vi "vacuum2.vi"() -> ()   [LabVIEW 2014, in "Panels.lvlib"]
uses:
  Panels.lvlib
  CSlibraries-extern/DimLVEvent/DimIndicators/DimIndicators.lvlib
  CS_Core/CSSystem/CoreLib/CoreLib.lvlib
  CSlibraries/UtilityLib/UtilityLib.valueStatus.ctl
  CSlibraries/UtilityLib/UtilityLib.lvlib
  CS_Core/CSSystem/CoreLib/CoreLib.short 2 byte array.vi
  Instance           1 15Saved   vacuum2 .vi
  Instance           2 15Saved   vacuum2 .vi
  Instance           3 15Saved   vacuum2 .vi
  Instance           4 15Saved   vacuum2 .vi
  Instance           5 15Saved   vacuum2 .vi
  CSlibraries-extern/DimLVEvent/LVDimInterface/LVDimInterface.lvlib
  CS_Core/CSSystem/CoreLib/CoreLib.string 2 byte array.vi
  CS_Core/BaseProcess/BaseProcess.descriptor string definition.ctl
  CS_Core/BaseProcess/BaseProcess.lvlib
  CS_Core/CSSystem/CoreDefs/CoreDefs.rawDataType.ctl
  CS_Core/CSSystem/CoreDefs/CoreDefs.call_type.ctl
  CSlibraries-extern/DimLVEvent/DimIndicators/DimIndicators.numericType.ctl
  CSlibraries-extern/DimLVEvent/DimIndicators/DimIndicators.numericArrayType.ctl
  CSlibraries-extern/DimLVEvent/DimIndicators/DimIndicators.anyType.ctl
panel:
  out "i ref out":refnum<vi>
  out "i ref out":refnum<vi>
  in  "BOB2TISout_MonData":T1
  in  "BOB2TISin_MonData":T1
  out "BOB2TIS":bool
  in  "FVCPIR_MonData":T1={"data"=inf, "no link"=FALSE, "quality"=1, "timeStamp"=3265900746.554}
  out "FVCPIR":dbl=inf format="%.2e"
  out "LHeLevel":dbl=inf format="%.4f"
  out "LN2Level":dbl=inf format="%.4f"
  in  "LN2Level_MonData":T1={"data"=inf, "no link"=FALSE, "quality"=1, "timeStamp"=3265900746.538}
  in  "LHeLevel_MonData":T1={"data"=inf, "no link"=FALSE, "quality"=1, "timeStamp"=3265900746.554}
  in  "call cluster in":T2={"Object"="", "Selector"="", "CallType"=enum."synchronous", "Async Object"="", "Async Selector"="", "Data Descriptor"="", "Data"=[], "Error #"=0, "Expire"=0}
  in  "ReasonForLocking_SetData":T5
  in  "call cluster in":T2={"Object"="", "Selector"="", "CallType"=enum."synchronous", "Async Object"="", "Async Selector"="", "Data Descriptor"="", "Data"=[], "Error #"=0, "Expire"=0}
  in  "Reason for locking":string
  in  "BOB6_MCP_SetData":T6={"data"=[0.0, 0.0, 0.0, 0.0], "no link"=FALSE, "quality"=1, "timeStamp"=3270208307.575}
  in  "BOB6_Pho_SetData":T6={"data"=[0.0, 0.0, 0.0, 0.0], "no link"=FALSE, "quality"=1, "timeStamp"=3270208307.575}
  in  "BOB5_MCP_SetData":T6={"data"=[0.0, 0.0, 0.0, 0.0], "no link"=FALSE, "quality"=1, "timeStamp"=3270208307.575}
  in  "BOB5_Pho_SetData":T6={"data"=[0.0, 0.0, 0.0, 0.0], "no link"=FALSE, "quality"=1, "timeStamp"=3270208307.575}
  in  "BOB3_MCP_SetData":T6={"data"=[0.0, 0.0, 0.0, 0.0], "no link"=FALSE, "quality"=1, "timeStamp"=3270208307.575}
  in  "BOB3_Pho_SetData":T6={"data"=[0.0, 0.0, 0.0, 0.0], "no link"=FALSE, "quality"=1, "timeStamp"=3270208307.591}
  in  "CB5SAFE_MonData":T1
  in  "FVAPIR_MonData":T1={"data"=inf, "no link"=FALSE, "quality"=1, "timeStamp"=3265900746.538}
  in  "FVBPIR_MonData":T1={"data"=inf, "no link"=FALSE, "quality"=1, "timeStamp"=3265900746.554}
  in  "BOB6_Pho_MonData":T1={"data"=inf, "no link"=FALSE, "quality"=1, "timeStamp"=3265900746.538}
  in  "BOB5PIR_MonData":T1={"data"=inf, "no link"=FALSE, "quality"=1, "timeStamp"=3265900746.538}
  in  "PT1PEN_MonData":T1={"data"=inf, "no link"=FALSE, "quality"=1, "timeStamp"=3265900746.538}
  in  "PT1PIR_MonData":T1={"data"=inf, "no link"=FALSE, "quality"=1, "timeStamp"=3265900746.522}
  in  "BOB6_MCP_MonData":T1={"data"=inf, "no link"=FALSE, "quality"=1, "timeStamp"=3265900746.554}
  in  "PT2PIR_MonData":T1={"data"=inf, "no link"=FALSE, "quality"=1, "timeStamp"=3265900746.569}
  in  "PT2PEN_MonData":T1={"data"=inf, "no link"=FALSE, "quality"=1, "timeStamp"=3265900746.554}
  in  "PTLN2PIR_MonData":T1={"data"=inf, "no link"=FALSE, "quality"=1, "timeStamp"=3265900746.538}
  in  "CBLN2PIR_MonData":T1={"data"=inf, "no link"=FALSE, "quality"=1, "timeStamp"=3265900746.569}
  in  "BOB2PEN_MonData":T1={"data"=inf, "no link"=FALSE, "quality"=1, "timeStamp"=3265900746.554}
  in  "BOB2PIR_MonData":T1={"data"=inf, "no link"=FALSE, "quality"=1, "timeStamp"=3265900746.538}
  in  "BOB3PEN_MonData":T1={"data"=inf, "no link"=FALSE, "quality"=1, "timeStamp"=3265900746.569}
  in  "BOB5PEN_MonData":T1={"data"=inf, "no link"=FALSE, "quality"=1, "timeStamp"=3265900746.569}
  in  "BOB5_Pho_MonData":T1={"data"=inf, "no link"=FALSE, "quality"=1, "timeStamp"=3265900746.538}
  in  "BOB5_MCP_MonData":T1={"data"=inf, "no link"=FALSE, "quality"=1, "timeStamp"=3265900746.585}
  in  "BOB4PIR_MonData":T1={"data"=inf, "no link"=FALSE, "quality"=1, "timeStamp"=3265900746.538}
  in  "BOB4PEN_MonData":T1={"data"=inf, "no link"=FALSE, "quality"=1, "timeStamp"=3265900746.554}
  in  "CB3PEN_MonData":T1={"data"=inf, "no link"=FALSE, "quality"=1, "timeStamp"=3265900746.569}
  in  "CB2PEN_MonData":T1={"data"=inf, "no link"=FALSE, "quality"=1, "timeStamp"=3265900746.522}
  in  "CB1PEN_MonData":T1={"data"=inf, "no link"=FALSE, "quality"=1, "timeStamp"=3265900746.538}
  in  "BOB3_Pho_MonData":T1={"data"=inf, "no link"=FALSE, "quality"=1, "timeStamp"=3265900746.6}
  in  "BOB3_MCP_MonData":T1={"data"=inf, "no link"=FALSE, "quality"=1, "timeStamp"=3265900746.585}
  in  "BOB3PIR_MonData":T1={"data"=inf, "no link"=FALSE, "quality"=1, "timeStamp"=3265900746.569}
  out "FVAPIR":dbl=inf format="%.2e"
  out "FVBPIR":dbl=inf format="%.2e"
  out "BOB6_Pho":dbl=inf format="%.3f"
  out "BOB6_MCP":dbl=inf format="%.3f"
  out "PT1PIR":dbl=inf format="%.2e"
  out "PT1PEN":dbl=inf format="%.2e"
  out "PT2PIR":dbl=inf format="%.2e"
  out "PT2PEN":dbl=inf format="%.2e"
  out "BOB5_Pho":dbl=inf format="%.3f"
  out "BOB5_MCP":dbl=inf format="%.3f"
  out "BOB5PIR":dbl=inf format="%.2e"
  out "BOB5PEN":dbl=inf format="%.2e"
  out "BOB4PIR":dbl=inf format="%.2e"
  out "BOB4PEN":dbl=inf format="%.2e"
  out "CB3PEN":dbl=inf format="%.2e"
  out "CB2PEN":dbl=inf format="%.2e"
  out "CB1PEN":dbl=inf format="%.2e"
  out "BOB3_Pho":dbl=inf format="%.3f"
  out "BOB3_MCP":dbl=inf format="%.3f"
  out "BOB3PIR":dbl=inf format="%.2e"
  out "BOB3PEN":dbl=inf format="%.2e"
  out "BOB2PIR":dbl=inf format="%.2e"
  out "BOB2PEN":dbl=inf format="%.2e"
  out "PTLN2PIR":dbl=inf format="%.2e"
  out "CBLN2PIR":dbl=inf format="%.2e"
  in  "LASFVAout_MonData":T1
  in  "LASFVBout_MonData":T1
  in  "LASGVSout_MonData":T1
  in  "BOB2FCout_MonData":T1
  in  "BOB2FVAout_MonData":T1
  in  "BOB2FVBout_MonData":T1
  in  "BOB2GVPout_MonData":T1
  in  "BOB2GVSout_MonData":T1
  in  "BOB2TPout_MonData":T1
  in  "TSTGVSout_MonData":T1
  in  "TSTTPout_MonData":T1
  in  "TSTFVAout_MonData":T1
  in  "TSTFVBout_MonData":T1
  in  "BOB3GVSout_MonData":T1
  in  "BOB3GVPout_MonData":T1
  in  "BOB3TPout_MonData":T1
  in  "BOB3FCout_MonData":T1
  in  "BOB3MCPout_MonData":T1
  in  "BOB3FVAout_MonData":T1
  in  "BOB3FVBout_MonData":T1
  in  "CBFVAout_MonData":T1
  in  "CBFVBout_MonData":T1
  in  "CBFVCout_MonData":T1
  in  "CB1TPout_MonData":T1
  in  "CB2TPout_MonData":T1
  in  "CB3TPout_MonData":T1
  in  "CB4TPout_MonData":T1
  in  "CB5GVSout_MonData":T1
  in  "BOB4GVSout_MonData":T1
  in  "BOB4GVPout_MonData":T1
  in  "BOB4TPout_MonData":T1
  in  "BOB4BETAout_MonData":T1
  in  "BOB4FVAout_MonData":T1
  in  "BOB4FVBout_MonData":T1
  in  "BOB5GVSout_MonData":T1
  in  "BOB5GVPout_MonData":T1
  in  "BOB5TPout_MonData":T1
  in  "BOB5FCout_MonData":T1
  in  "BOB5MCPout_MonData":T1
  in  "BOB5FVAout_MonData":T1
  in  "BOB5FVBout_MonData":T1
  in  "PT1GVPout_MonData":T1
  in  "PT1TPout_MonData":T1
  in  "PT1FVAout_MonData":T1
  in  "PT1FVBout_MonData":T1
  in  "PT2GVPout_MonData":T1
  in  "PT2TPout_MonData":T1
  in  "PT2FVAout_MonData":T1
  in  "PT2FVBout_MonData":T1
  in  "BOB2lock_SetData":T1
  in  "BOB3lock_SetData":T1
  in  "BOB4lock_SetData":T1
  in  "BOB5lock_SetData":T1
  in  "TSTlock_SetData":T1
  in  "CBlock_SetData":T1
  in  "PTlock_SetData":T1
  in  "LASlock_SetData":T1
  in  "PT2FVBin_MonData":T1
  in  "PT2FVAin_MonData":T1
  in  "PT2TPin_MonData":T1
  in  "PT2GVPin_MonData":T1
  in  "PT1FVBin_MonData":T1
  in  "PT1FVAin_MonData":T1
  in  "PT1TPin_MonData":T1
  in  "PT1GVPin_MonData":T1
  in  "BOB5FVBin_MonData":T1
  in  "BOB5FVAin_MonData":T1
  in  "BOB5MCPin_MonData":T1
  in  "BOB5FCin_MonData":T1
  in  "BOB5TPin_MonData":T1
  in  "BOB5GVPin_MonData":T1
  in  "BOB5GVSin_MonData":T1
  in  "BOB4FVBin_MonData":T1
  in  "BOB4FVAin_MonData":T1
  in  "BOB4BETAin_MonData":T1
  in  "BOB4TPin_MonData":T1
  in  "BOB4GVPin_MonData":T1
  in  "BOB4GVSin_MonData":T1
  in  "CB5GVSin_MonData":T1
  in  "CB4TPin_MonData":T1
  in  "CB3TPin_MonData":T1
  in  "CB2TPin_MonData":T1
  in  "CB1TPin_MonData":T1
  in  "CBFVCin_MonData":T1
  in  "CBFVBin_MonData":T1
  in  "CBFVAin_MonData":T1
  in  "BOB3FVBin_MonData":T1
  in  "BOB3FVAin_MonData":T1
  in  "BOB3MCPin_MonData":T1
  in  "BOB3FCin_MonData":T1
  in  "BOB3TPin_MonData":T1
  in  "BOB3GVPin_MonData":T1
  in  "BOB3GVSin_MonData":T1
  in  "TSTFVBin_MonData":T1
  in  "TSTFVAin_MonData":T1
  in  "TSTTPin_MonData":T1
  in  "TSTGVSin_MonData":T1
  in  "BOB2TPin_MonData":T1
  out "TSTlock":bool
  out "BOB3lock":bool
  out "BOB6FC":bool
  out "BOB6MCP":bool=TRUE
  out "BOB3MCP":bool
  out "BOB3FC":bool
  out "BOB2FC":bool
  out "LASlock":bool
  out "BOB2lock":bool
  out "BOB5MCP":bool
  out "BOB5FC":bool
  out "BOB4BETA":bool
  out "CBlock":bool
  out "PTlock":bool
  out "BOB5lock":bool
  out "BOB4lock":bool
  out "LASGVS":bool
  out "TSTGVS":bool
  out "BOB2GVS":bool
  out "BOB3GVS":bool
  out "BOB4GVS":bool
  out "BOB5GVS":bool
  out "BOB2GVP":bool
  out "BOB3GVP":bool
  out "CB5GVS":bool
  out "BOB4GVP":bool
  out "BOB5GVP":bool
  out "PT1GVP":bool
  out "PT2GVP":bool
  out "LASFVA":bool
  out "LASFVB":bool
  out "BOB2FVA":bool
  out "BOB2FVB":bool
  out "TSTFVA":bool
  out "TSTFVB":bool
  out "BOB3FVA":bool
  out "BOB3FVB":bool
  out "CBFVA":bool
  out "CBFVC":bool
  out "CBFVB":bool
  out "BOB4FVA":bool
  out "BOB4FVB":bool
  out "BOB5FVA":bool
  out "BOB5FVB":bool
  out "PT1FVA":bool
  out "PT1FVB":bool
  out "PT2FVA":bool
  out "PT2FVB":bool
  out "CB1TP":bool
  out "BOB3TP":bool
  out "TSTTP":bool
  out "CB2TP":bool
  out "BOB2TP":bool
  out "CB5SAFE":bool=TRUE
  out "BOB5TP":bool
  out "PT2TP":bool
  out "BOB4TP":bool
  out "PT1TP":bool
  out "CB4TP":bool
  out "CB3TP":bool
  in  "BOB2GVSin_MonData":T1
  in  "BOB2GVPin_MonData":T1
  out "i ref out":refnum<vi>
  in  "BOB2FVAin_MonData":T1
  in  "BOB2FCin_MonData":T1
  in  "LASGVSin_MonData":T1
  in  "LASFVBin_MonData":T1
  in  "LASFVAin_MonData":T1
  in  "BOB2FVBin_MonData":T1
  out "PT2FVBen":bool
  out "PT2FVAen":bool
  out "PT1FVBen":bool
  out "PT1FVAen":bool
  out "BOB5FVBen":bool
  out "BOB5FVAen":bool
  out "BOB4FVBen":bool
  out "BOB4FVAen":bool
  out "BOB3FVBen":bool
  out "BOB3FVAen":bool
  out "TSTFVBen":bool
  out "BOB2FVBen":bool
  out "TSTFVAen":bool
  out "BOB2FVAen":bool
  out "LASFVBen":bool
  out "LASFVAen":bool
  out "CBFVCen":bool
  out "CBFVBen":bool
  out "CBFVAen":bool
  out "PT2GVPen":bool
  out "PT1GVPen":bool
  out "BOB5GVPen":bool
  out "BOB4GVPen":bool
  out "BOB3GVPen":bool
  out "BOB2GVPen":bool
  out "BOB5GVSen":bool
  out "BOB4GVSen":bool
  out "BOB3GVSen":bool
  out "BOB2GVSen":bool
  out "LASGVSen":bool
  out "TSTGVSen":bool
  out "BOB2TPen":bool
  out "TSTTPen":bool
  out "BOB3TPen":bool
  out "BOB4TPen":bool
  out "BOB5TPen":bool
  out "PT1TPen":bool
  out "PT2TPen":bool
  out "CB1TPen":bool
  out "CB5GVSen":bool
  # "voltage"
  # "V"
  # "voltage"
  # "V"
  # "CB5SAFE"
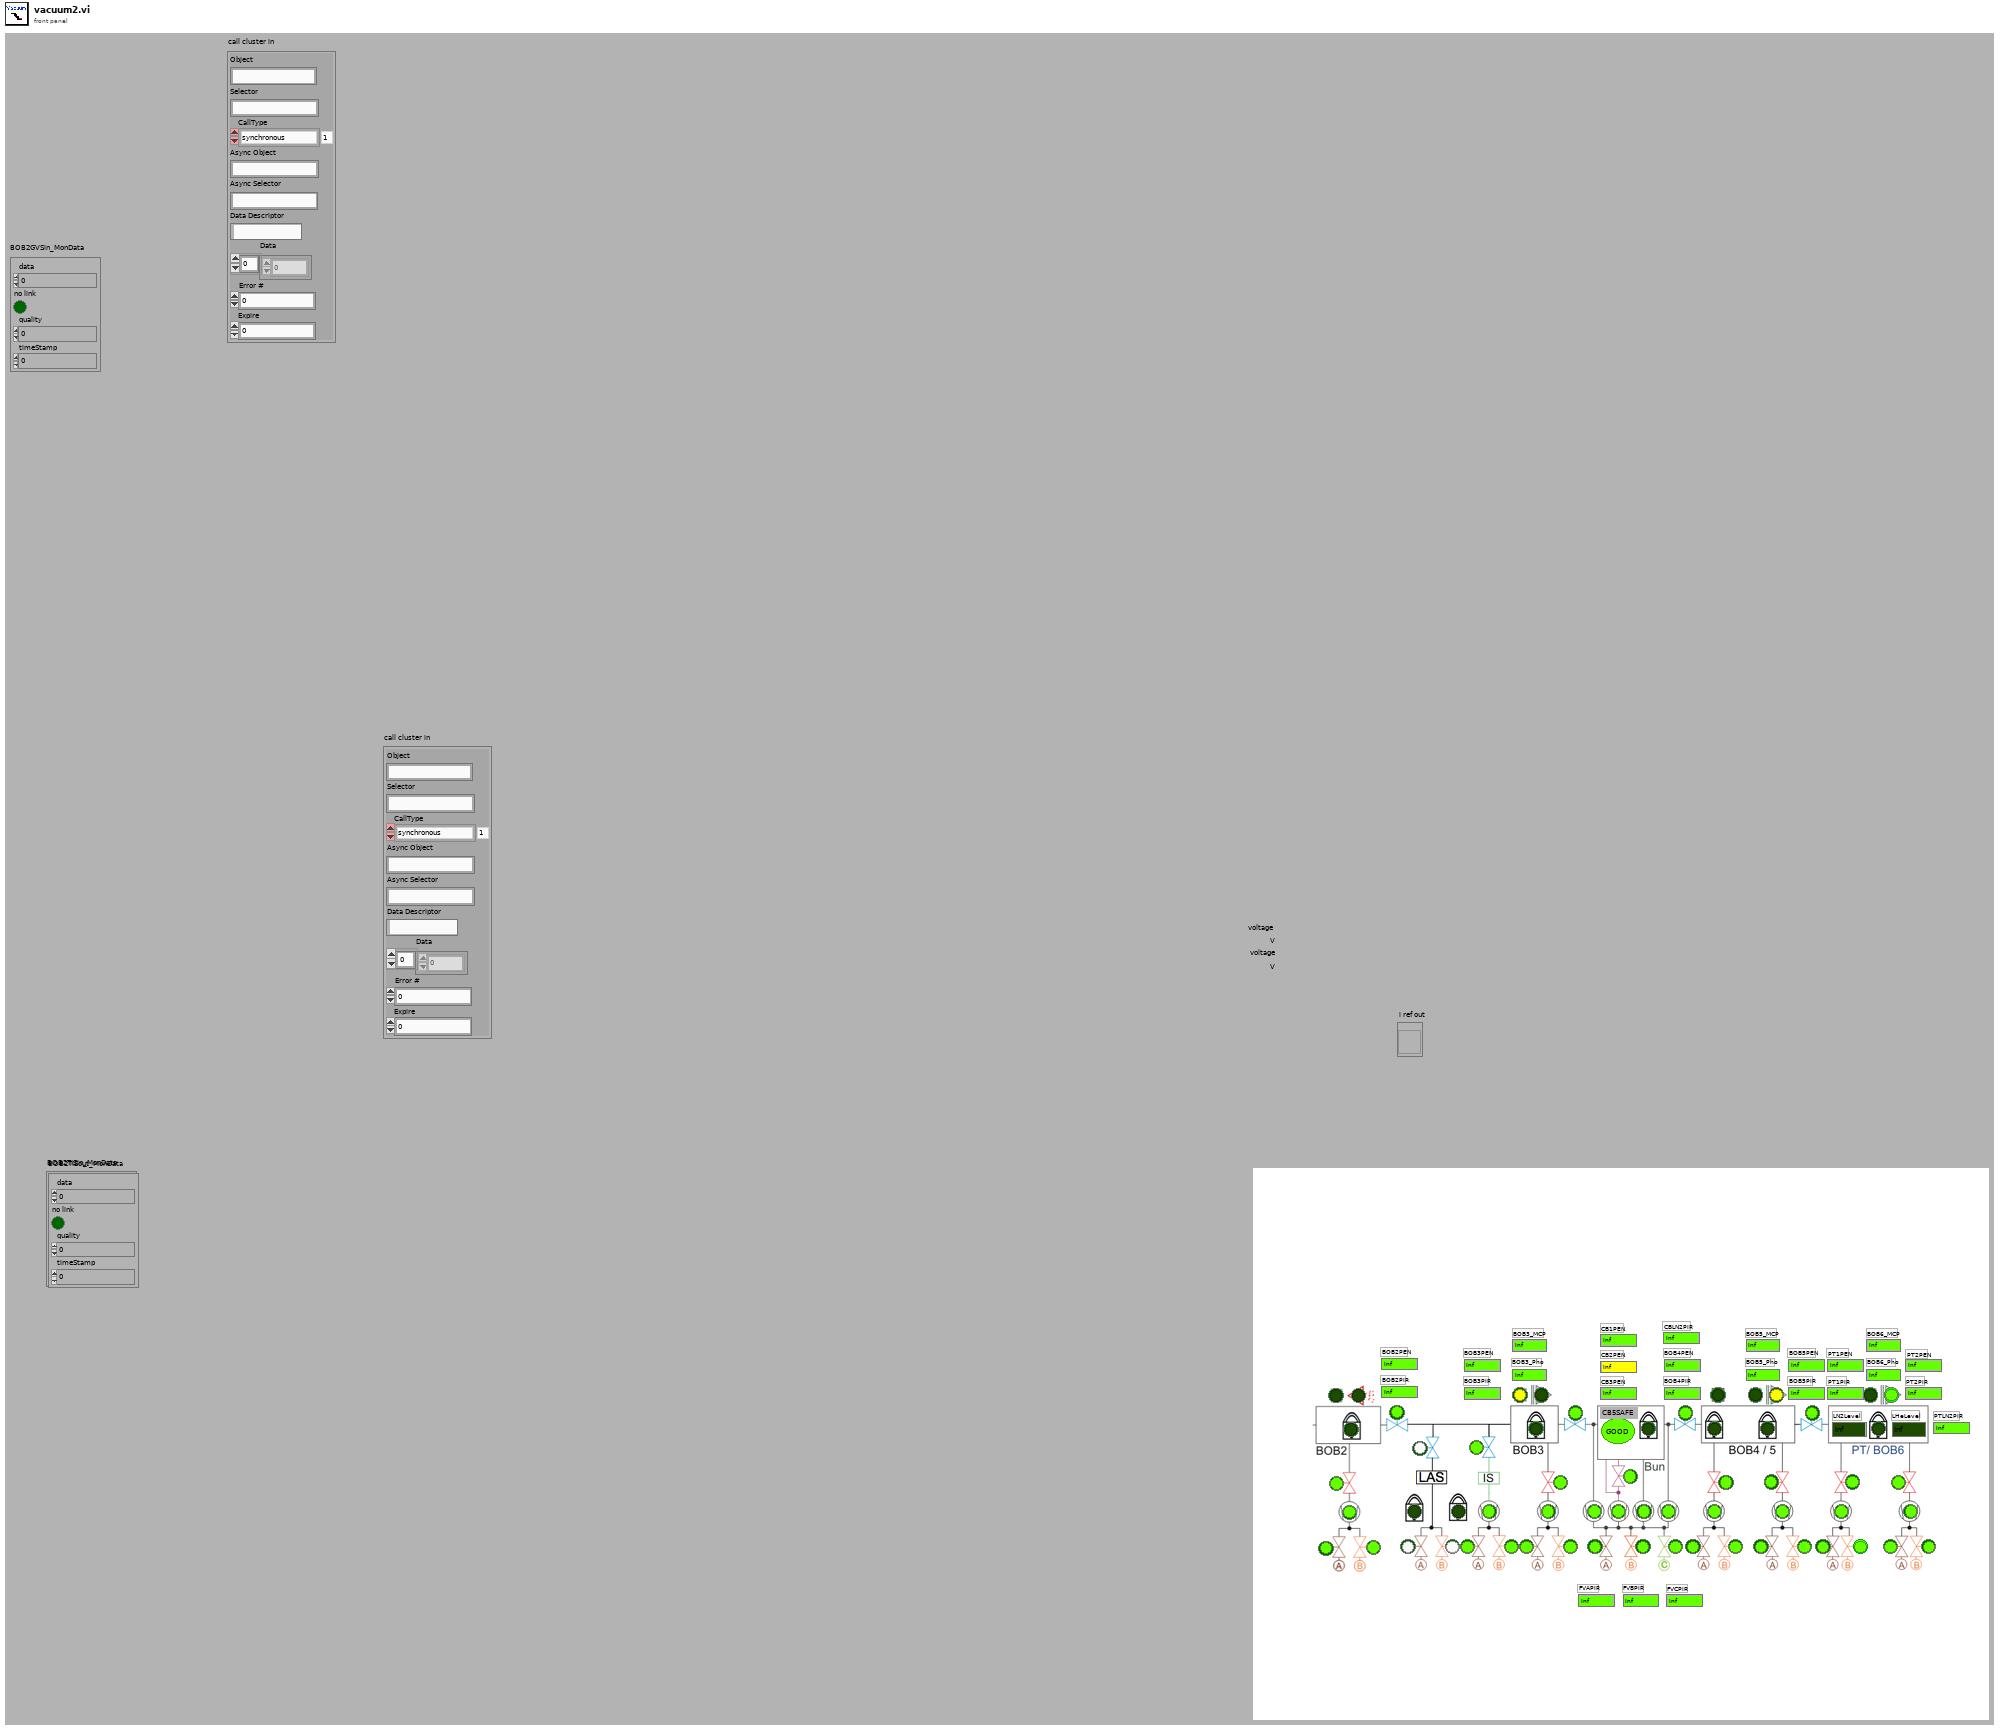
[diagram p1: front panel]
types:
  T1 = typedef "DimIndicators.lvlib/DimIndicators.numericType.ctl" = cluster{"data":dbl, "no link":bool, "quality":i32, "timeStamp":dbl}
  T2 = typedef "CoreDefs.call_type.ctl" = cluster{"Object":string, "Selector":string, "CallType":enum16{"simple", "synchronous", "asynchronous"}, "Async Object":string, "Async Selector":string, "Data Descriptor":T3, "Data":T4, "Error #":i32, "Expire":u32}
  T3 = typedef "BaseProcess.lvlib/BaseProcess.descriptor string definition.ctl" = string
  T4 = typedef "CoreDefs.rawDataType.ctl" = i8[]
  T5 = typedef "DimIndicators.lvlib/DimIndicators.anyType.ctl" = cluster{"data":string, "no link":bool, "quality":i32, "timeStamp":dbl}
  T6 = typedef "DimIndicators.lvlib/DimIndicators.numericArrayType.ctl" = cluster{"data":dbl[], "no link":bool, "quality":i32, "timeStamp":dbl}
  T7 = typedef "UtilityLib.lvlib/UtilityLib.valueStatus.ctl" = enum16{"no info available", "stand by/off", "on", "warning", "alarm/malfunction", "not implemented", "user action required", "important information", "system default", "control default", "indicator default", "button default"}
  T8 = cluster{"data":i16, "no link":bool, "quality":i32, "timeStamp":dbl}
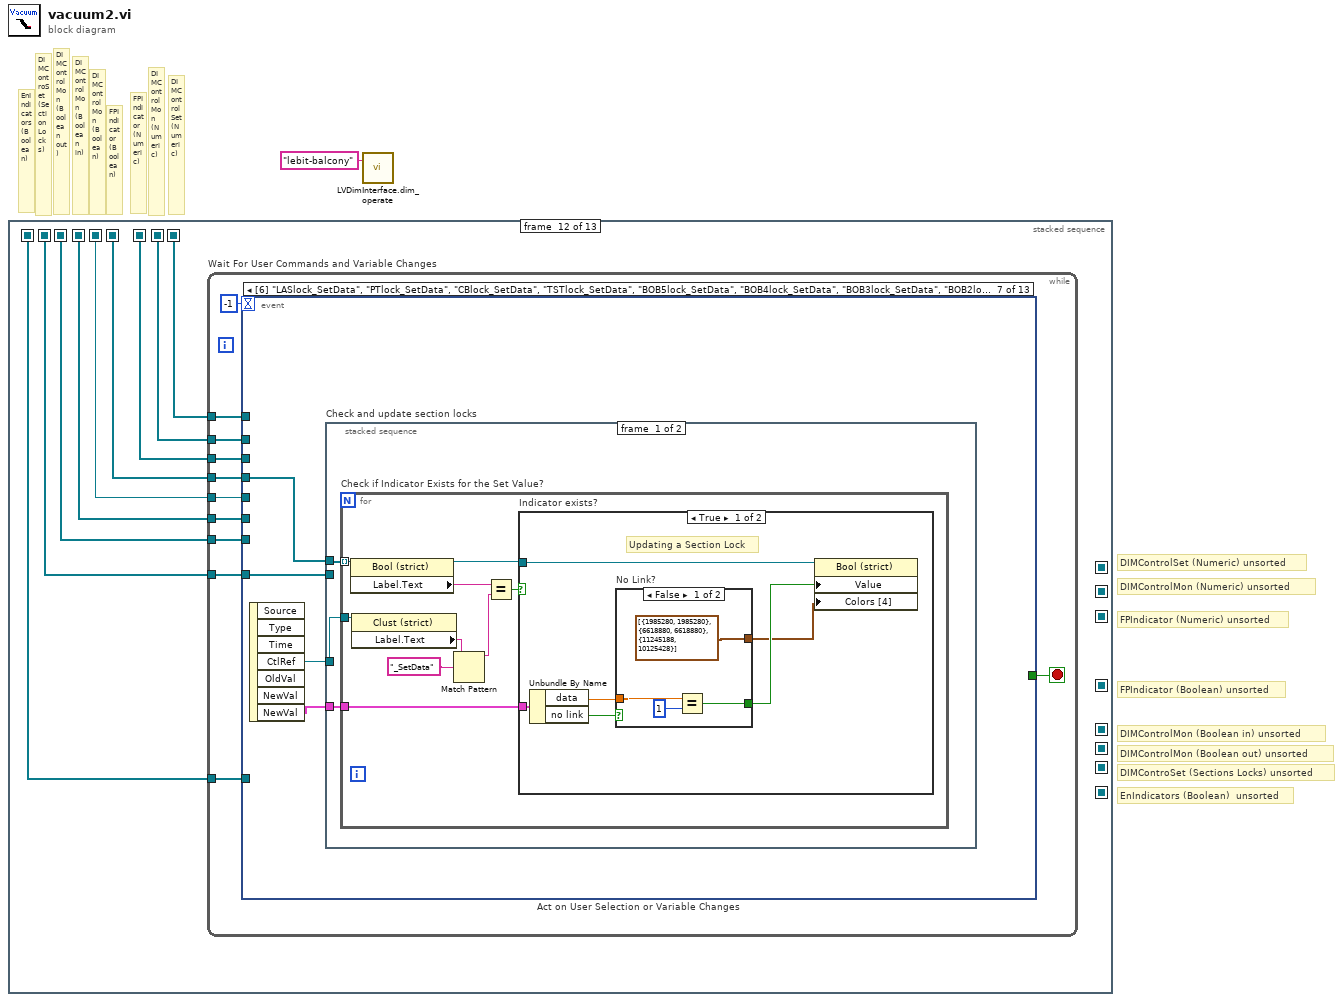
[diagram p0: block diagram]
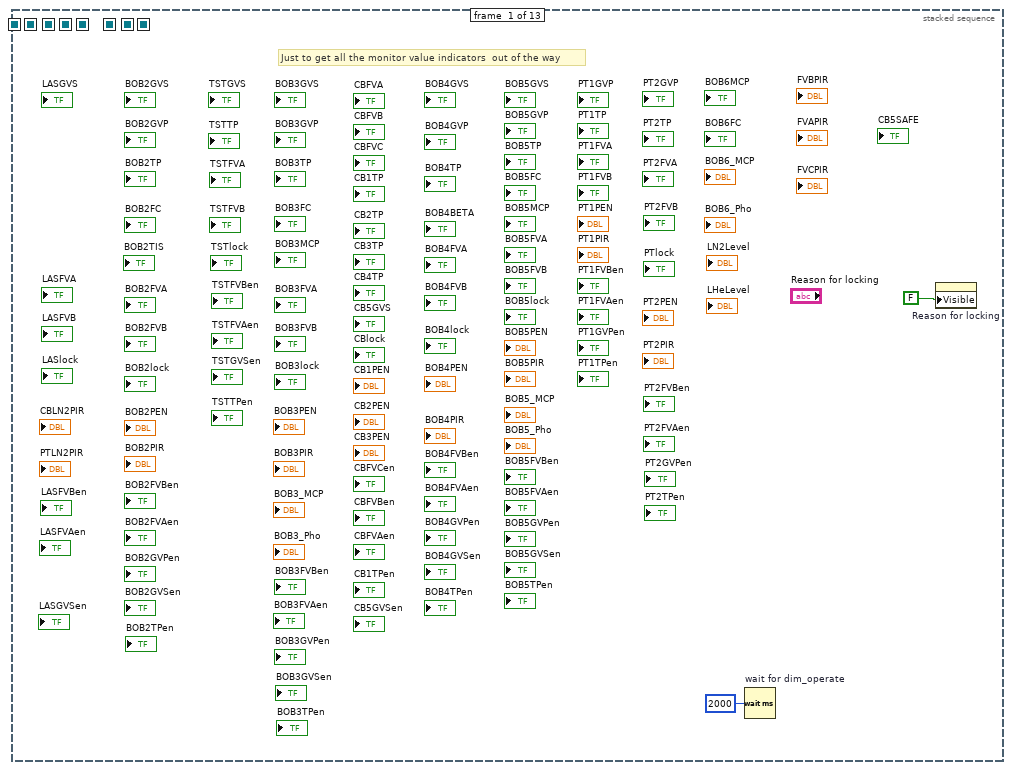
[diagram p2: hidden frame]
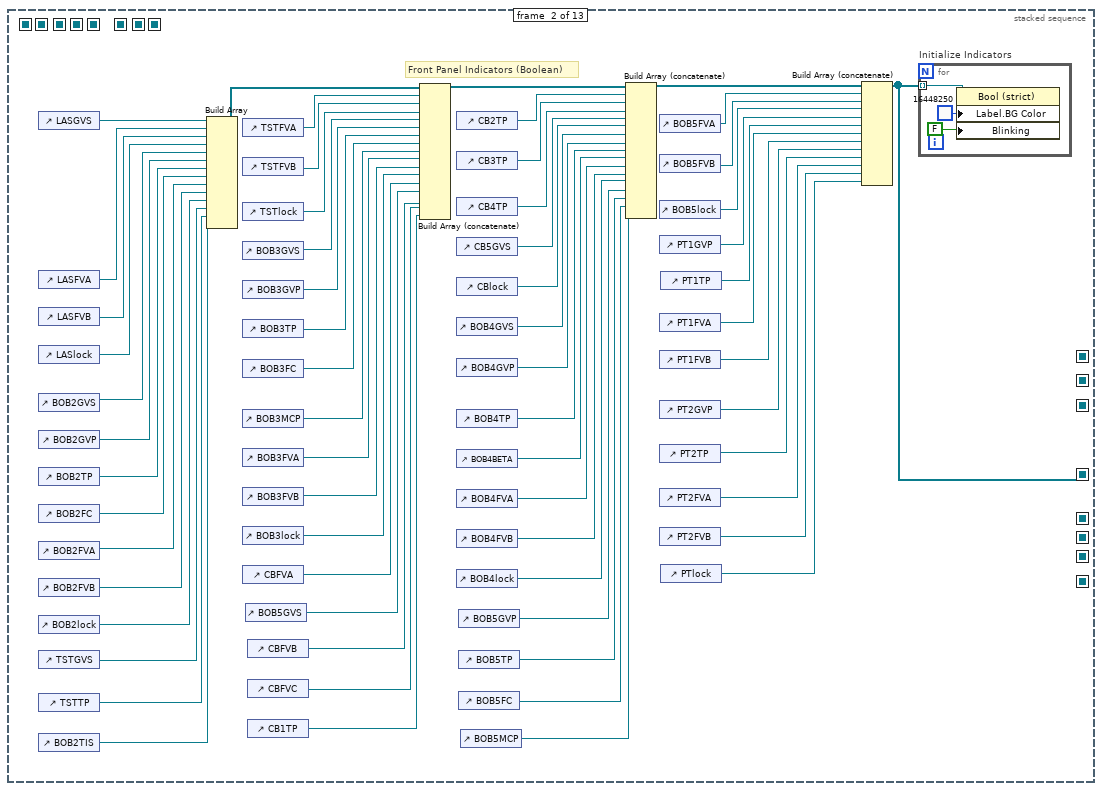
[diagram p3: hidden frame]
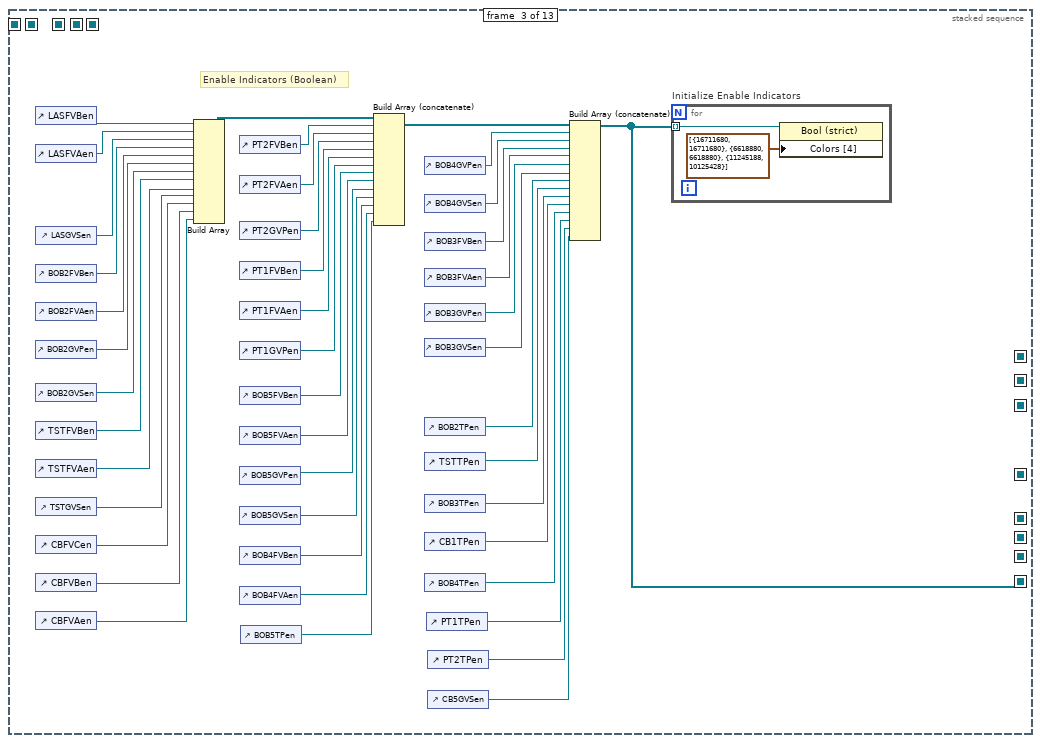
[diagram p4: hidden frame]
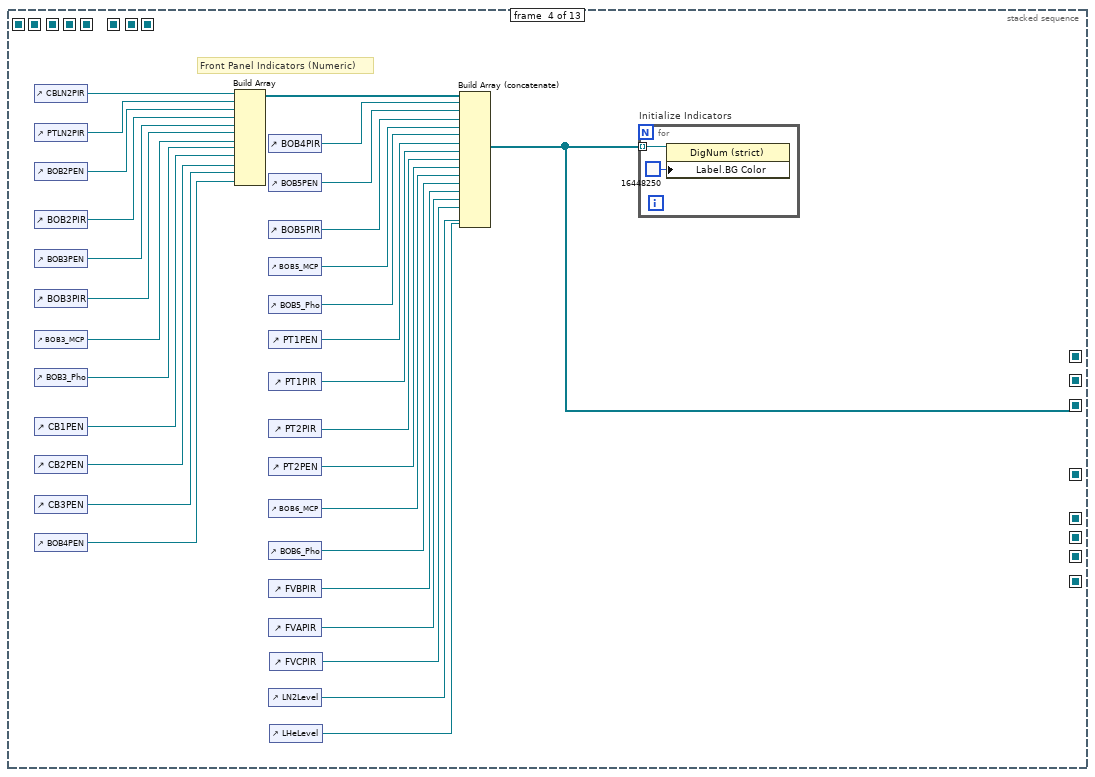
[diagram p5: hidden frame]
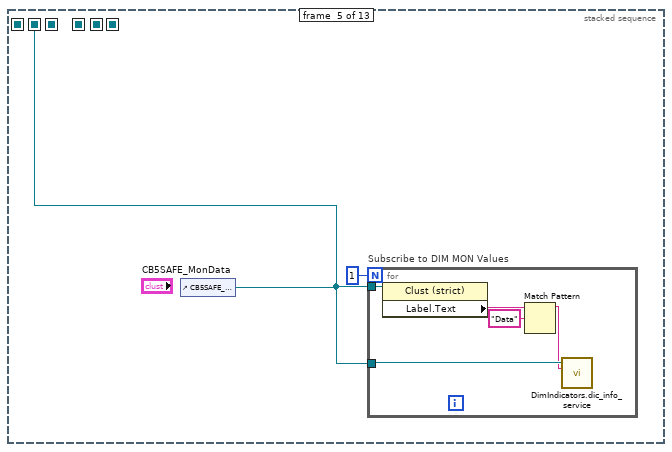
[diagram p6: hidden frame]
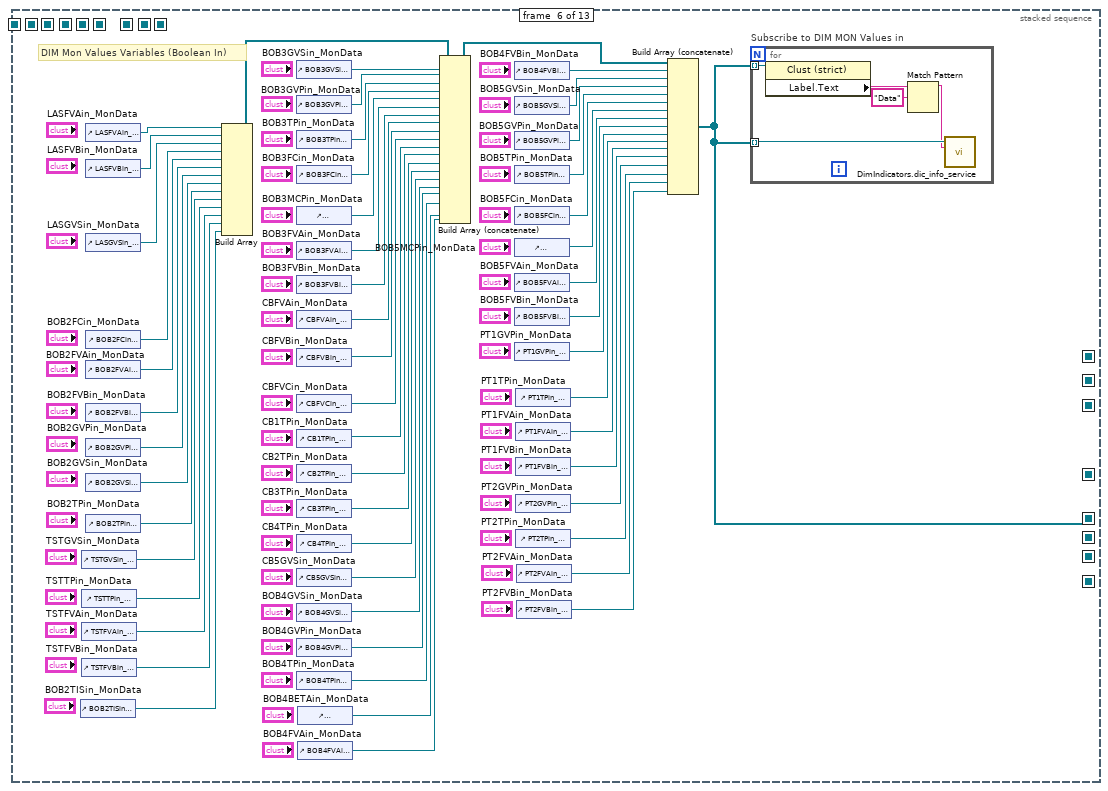
[diagram p7: hidden frame]
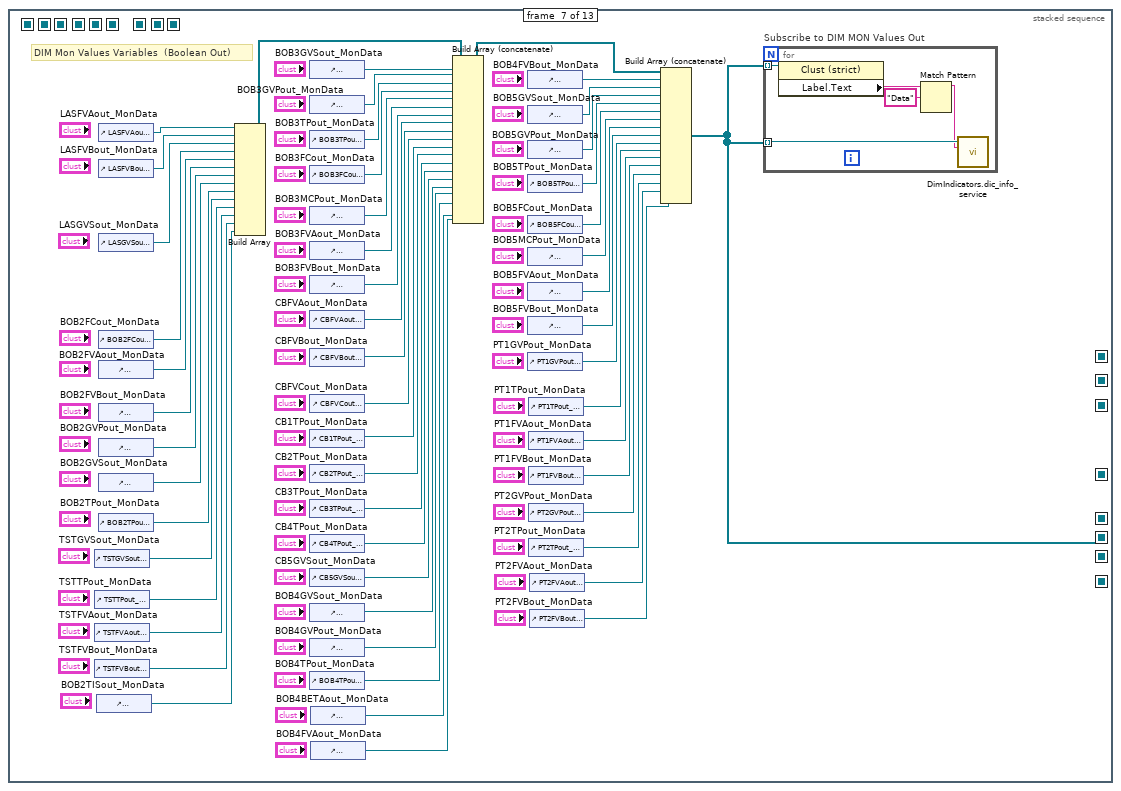
[diagram p8: hidden frame]
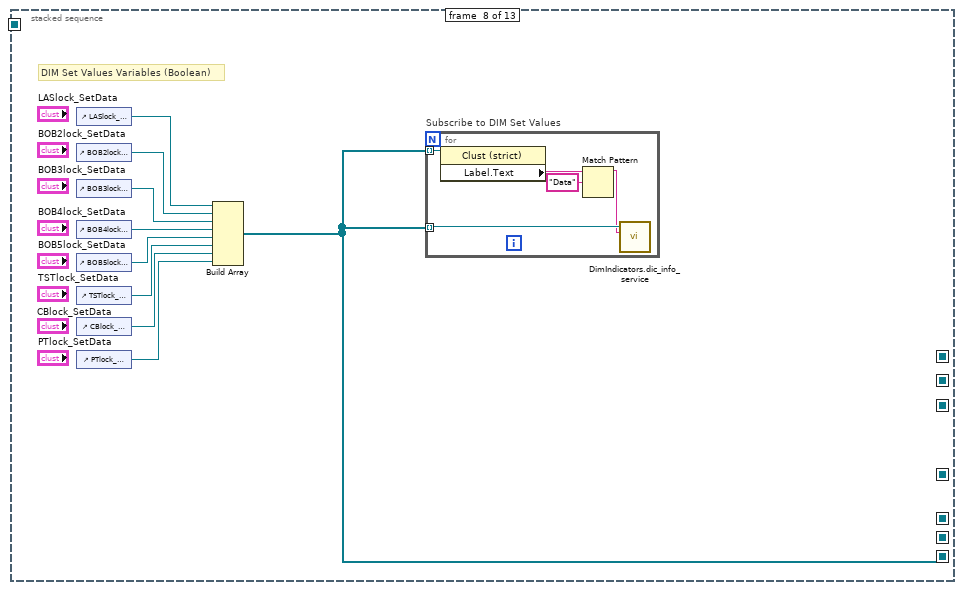
[diagram p9: hidden frame]
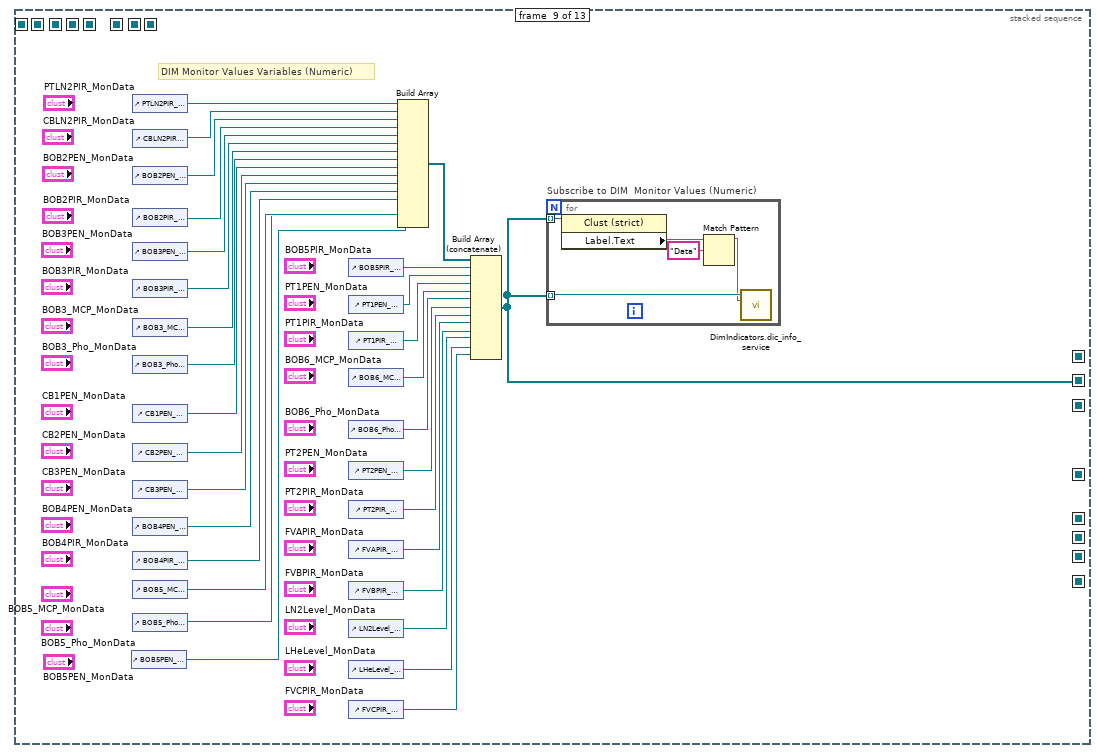
[diagram p10: hidden frame]
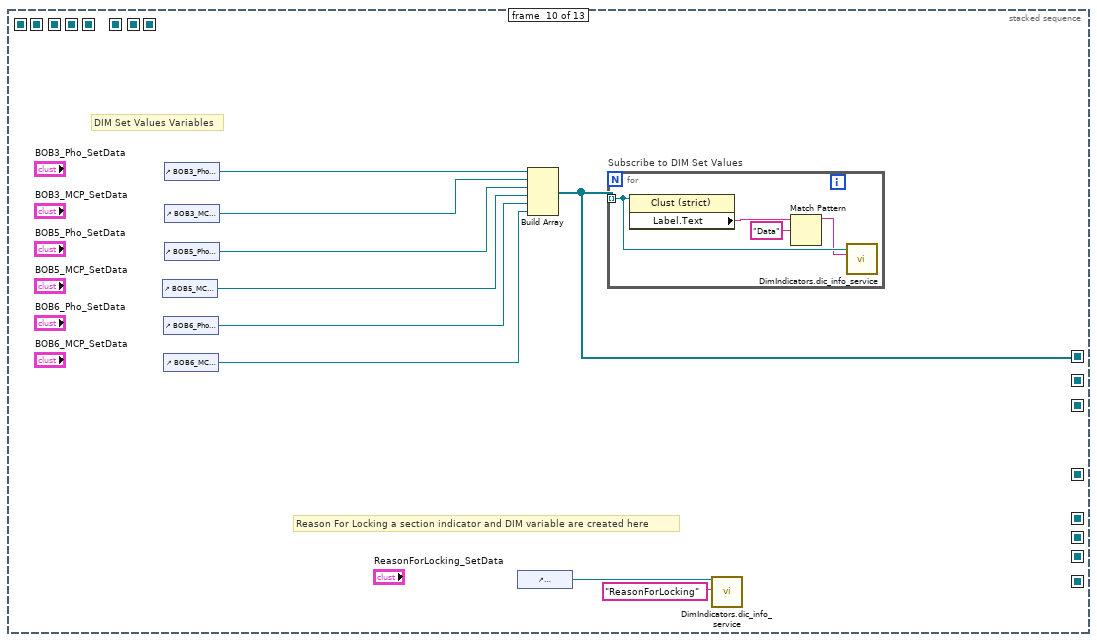
[diagram p11: hidden frame]
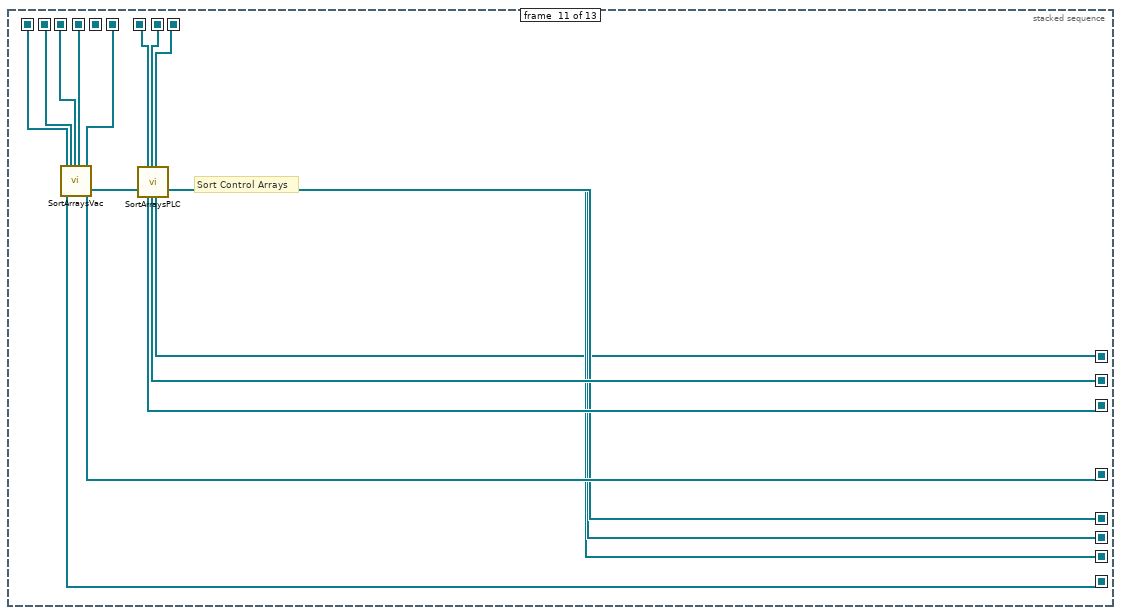
[diagram p12: hidden frame]
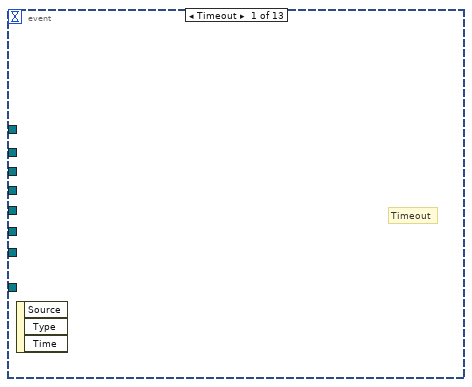
[diagram p13: hidden frame]
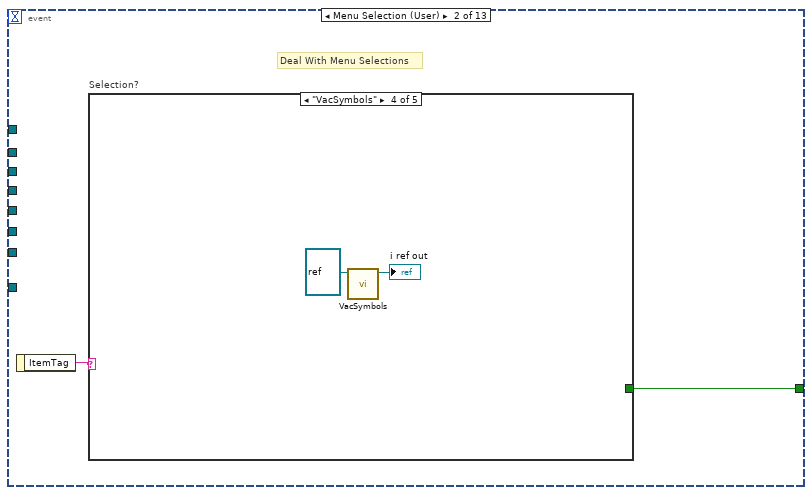
[diagram p14: hidden frame]
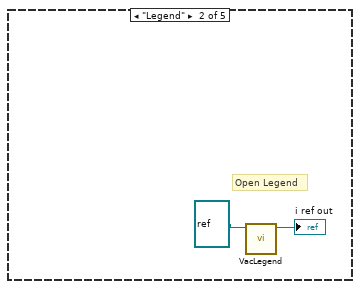
[diagram p16: hidden frame]
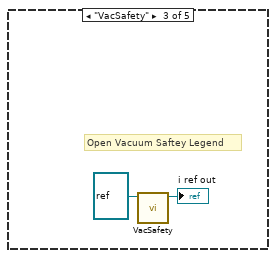
[diagram p17: hidden frame]
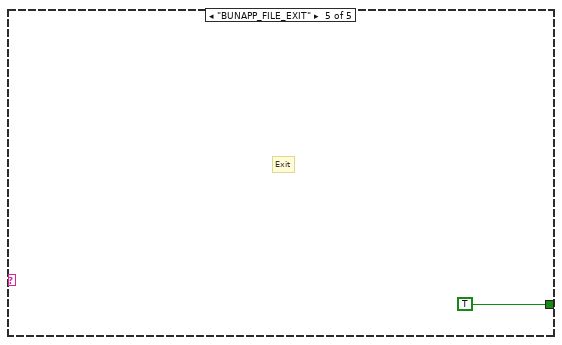
[diagram p18: hidden frame]
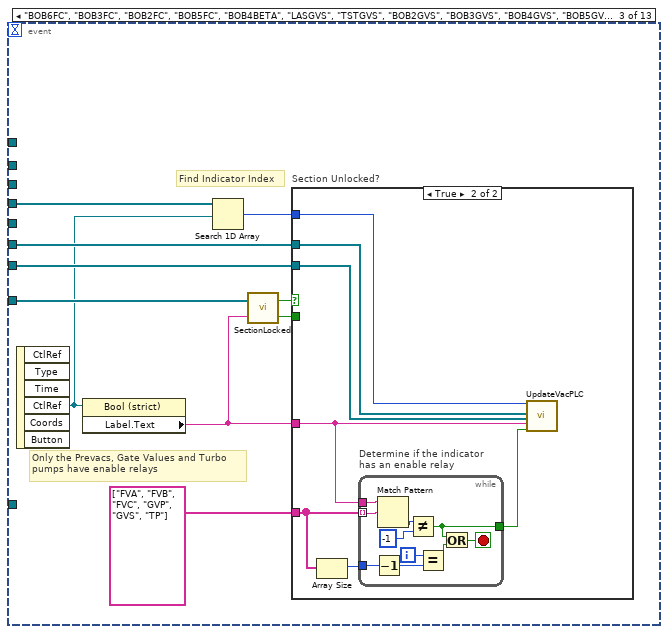
[diagram p19: hidden frame]
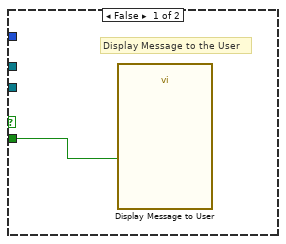
[diagram p20: hidden frame]
diagram:
  # "EnIndicators (Boolean)"
  # "EnIndicators (Boolean)  unsorted"
  # "DIMControlSet (Numeric)"
  # "DIMControlSet (Numeric) unsorted"
  # "DIMControlMon (Boolean)"
  # "DIMControlMon (Numeric) unsorted"
  # "DIMControlMon (Boolean out) unsorted"
  # "FPIndicator (Numeric) unsorted"
  # "DIMControSet (Sections Locks) unsorted"
  # "DIMControlMon (Boolean in) unsorted"
  # "FPIndicator (Boolean) unsorted"
  # "DIMControlMon (Numeric)"
  # "DIMControlMon (Boolean out)"
  # "FPIndicator (Numeric)"
  # "DIMControSet (Section Locks)"
  # "DIMControlMon (Boolean in)"
  # "FPIndicator (Boolean)"
  n1 = stacked-sequence {
    seq-local: [_ w7 _ _ _ _ _ _ _ _ _ _ _] -> [_ _ _ _ _ _ _ _ _ _ w346 _ _]
    seq-local: [_ _ _ _ _ w157 _ _ _ _ _ _ _] -> [_ _ _ _ _ _ _ _ _ _ w340 _ _]
    seq-local: [_ _ _ _ _ _ _ w269 _ _ _ _ _] -> [_ _ _ _ _ _ _ _ _ _ w338 _ _]
    seq-local: [_ _ _ w142 _ _ _ _ _ _ _ _ _] -> [_ _ _ _ _ _ _ _ _ _ w344 _ _]
    seq-local: [_ _ _ _ _ _ w215 _ _ _ _ _ _] -> [_ _ _ _ _ _ _ _ _ _ w339 _ _]
    seq-local: [_ _ _ _ _ _ _ _ w286 _ _ _ _] -> [_ _ _ _ _ _ _ _ _ _ w343 _ _]
    seq-local: [_ _ _ _ _ _ _ _ _ _ w341 _ _] -> [_ _ _ _ _ _ _ _ _ _ _ w354 w793]
    seq-local: [_ _ _ _ _ _ _ _ _ _ w337 _ _] -> [_ _ _ _ _ _ _ _ _ _ _ w351 w790]
    seq-local: [_ _ _ _ _ _ _ _ _ _ w335 _ _] -> [_ _ _ _ _ _ _ _ _ _ _ w352 w791]
    seq-local: [_ _ _ _ _ _ _ _ _ _ w336 _ _] -> [_ _ _ _ _ _ _ _ _ _ _ w353 w792]
    seq-local: [_ _ _ _ _ _ _ _ _ _ w342 _ _] -> [_ _ _ _ _ _ _ _ _ _ _ w355 _]
    seq-local: [_ _ _ _ _ _ _ _ _ _ w345 _ _] -> [_ _ _ _ _ _ _ _ _ _ _ w350 _]
    seq-local: [_ _ _ _ w147 _ _ _ _ _ _ _ _] -> [_ _ _ _ _ _ _ _ _ _ _ w349 w788]
    seq-local: [_ _ _ _ _ _ _ _ _ w320 _ _ _] -> [_ _ _ _ _ _ _ _ _ _ w334 _ _]
    seq-local: [_ _ _ _ _ _ _ _ _ _ w333 _ _] -> [_ _ _ _ _ _ _ _ _ _ _ w348 w789]
    seq-local: [_ _ w80 _ _ _ _ _ _ _ _ _ _] -> [_ _ _ _ _ _ _ _ _ _ w332 _ _]
    seq-local: [_ _ _ _ _ _ _ _ _ _ w331 _ _] -> [_ _ _ _ _ _ _ _ _ _ _ w347 _]
    frame #0 {
      # "Just to get all the monitor value indicators  out of the way"
      n2 = Wait (ms) "wait for dim_operate"(milliseconds to wait=u32 2000) -> ()  [unwired: 1 out]
      n3 = property on="Reason for locking" class="Str"("Visible"=FALSE) -> ()  [unwired: 2 in, 2 out]
    }
    frame #1 {
      # "Front Panel Indicators (Boolean)"
      # "Arrange references to all monitor-value related buttons into an array."
      n4 = control-ref of="LASGVS"() -> (w4:refnum<vi>)
      n5 = control-ref of="LASFVA"() -> (w65:refnum<vi>)
      n6 = control-ref of="LASFVB"() -> (w64:refnum<vi>)
      n7 = control-ref of="LASlock"() -> (w63:refnum<vi>)
      n8 = control-ref of="BOB2GVS"() -> (w62:refnum<vi>)
      n9 = control-ref of="BOB2GVP"() -> (w61:refnum<vi>)
      n10 = control-ref of="BOB2TP"() -> (w60:refnum<vi>)
      n11 = control-ref of="BOB2FC"() -> (w59:refnum<vi>)
      n12 = control-ref of="BOB2FVA"() -> (w58:refnum<vi>)
      n13 = control-ref of="BOB2FVB"() -> (w57:refnum<vi>)
      n14 = control-ref of="BOB2lock"() -> (w56:refnum<vi>)
      n15 = control-ref of="TSTGVS"() -> (w55:refnum<vi>)
      n16 = control-ref of="TSTTP"() -> (w54:refnum<vi>)
      n17 = control-ref of="BOB2TIS"() -> (w5:refnum<vi>)
      n18 = Build Array(w4, w65, w64, w63, w62, w61, w60, w59, w58, w57, w56, w55, w54, w5) -> (w53:refnum<vi>[])
      n19 = control-ref of="TSTFVA"() -> (w52:refnum<vi>)
      n20 = control-ref of="TSTFVB"() -> (w51:refnum<vi>)
      n21 = control-ref of="TSTlock"() -> (w50:refnum<vi>)
      n22 = control-ref of="BOB3GVS"() -> (w49:refnum<vi>)
      n23 = control-ref of="BOB3GVP"() -> (w48:refnum<vi>)
      n24 = control-ref of="BOB3TP"() -> (w47:refnum<vi>)
      n25 = control-ref of="BOB3FC"() -> (w46:refnum<vi>)
      n26 = control-ref of="BOB3MCP"() -> (w45:refnum<vi>)
      n27 = control-ref of="BOB3FVA"() -> (w44:refnum<vi>)
      n28 = control-ref of="BOB3FVB"() -> (w43:refnum<vi>)
      n29 = control-ref of="BOB3lock"() -> (w42:refnum<vi>)
      n30 = control-ref of="CBFVA"() -> (w41:refnum<vi>)
      n31 = control-ref of="BOB5GVS"() -> (w40:refnum<vi>)
      n32 = control-ref of="CBFVB"() -> (w39:refnum<vi>)
      n33 = control-ref of="CBFVC"() -> (w38:refnum<vi>)
      n34 = control-ref of="CB1TP"() -> (w37:refnum<vi>)
      n35 = Build Array (concatenate)(w53, w52, w51, w50, w49, w48, w47, w46, w45, w44, w43, w42, w41, w40, w39, w38, w37) -> (w36:refnum<vi>[])
      n36 = control-ref of="CB2TP"() -> (w35:refnum<vi>)
      n37 = control-ref of="CB3TP"() -> (w34:refnum<vi>)
      n38 = control-ref of="CB4TP"() -> (w33:refnum<vi>)
      n39 = control-ref of="CB5GVS"() -> (w32:refnum<vi>)
      n40 = control-ref of="CBlock"() -> (w31:refnum<vi>)
      n41 = control-ref of="BOB4GVS"() -> (w30:refnum<vi>)
      n42 = control-ref of="BOB4GVP"() -> (w29:refnum<vi>)
      n43 = control-ref of="BOB4TP"() -> (w28:refnum<vi>)
      n44 = control-ref of="BOB4BETA"() -> (w27:refnum<vi>)
      n45 = control-ref of="BOB4FVA"() -> (w26:refnum<vi>)
      n46 = control-ref of="BOB4FVB"() -> (w25:refnum<vi>)
      n47 = control-ref of="BOB4lock"() -> (w24:refnum<vi>)
      n48 = control-ref of="BOB5GVP"() -> (w23:refnum<vi>)
      n49 = control-ref of="BOB5TP"() -> (w22:refnum<vi>)
      n50 = control-ref of="BOB5FC"() -> (w21:refnum<vi>)
      n51 = control-ref of="BOB5MCP"() -> (w20:refnum<vi>)
      n52 = Build Array (concatenate)(w36, w35, w34, w33, w32, w31, w30, w29, w28, w27, w26, w25, w24, w23, w22, w21, w20) -> (w19:refnum<vi>[])
      n53 = control-ref of="BOB5FVA"() -> (w18:refnum<vi>)
      n54 = control-ref of="BOB5FVB"() -> (w17:refnum<vi>)
      n55 = control-ref of="BOB5lock"() -> (w16:refnum<vi>)
      n56 = control-ref of="PT1GVP"() -> (w15:refnum<vi>)
      n57 = control-ref of="PT1FVA"() -> (w14:refnum<vi>)
      n58 = control-ref of="PT1FVB"() -> (w13:refnum<vi>)
      n59 = control-ref of="PT2GVP"() -> (w12:refnum<vi>)
      n60 = control-ref of="PT2TP"() -> (w11:refnum<vi>)
      n61 = control-ref of="PT2FVA"() -> (w10:refnum<vi>)
      n62 = control-ref of="PT2FVB"() -> (w9:refnum<vi>)
      n63 = control-ref of="PT1TP"() -> (w6:refnum<vi>)
      n64 = control-ref of="PTlock"() -> (w8:refnum<vi>)
      n65 = Build Array (concatenate)(w19, w18, w17, w16, w15, w6, w14, w13, w12, w11, w10, w9, w8) -> (w7:refnum<vi>[])
      n66 = for "Initialize Indicators" {
        tunnel: w7 -> [w68] mode=indexing
        n67 = property class="Bool (strict)"(reference=w68, "Label.BG Color"=u32 16448250 ("Color Box"), "Blinking"=FALSE) -> ()  [unwired: 1 in, 2 out]
      }
    }
    frame #2 {
      # "Enable Indicators (Boolean)"
      n68 = control-ref of="LASFVBen"() -> (w69:refnum<vi>)
      n69 = control-ref of="LASFVAen"() -> (w70:refnum<vi>)
      n70 = control-ref of="LASGVSen"() -> (w111:refnum<vi>)
      n71 = control-ref of="BOB2FVBen"() -> (w110:refnum<vi>)
      n72 = control-ref of="BOB2FVAen"() -> (w109:refnum<vi>)
      n73 = control-ref of="BOB2GVPen"() -> (w108:refnum<vi>)
      n74 = control-ref of="BOB2GVSen"() -> (w107:refnum<vi>)
      n75 = control-ref of="TSTFVBen"() -> (w106:refnum<vi>)
      n76 = control-ref of="TSTFVAen"() -> (w105:refnum<vi>)
      n77 = control-ref of="TSTGVSen"() -> (w104:refnum<vi>)
      n78 = control-ref of="CBFVCen"() -> (w103:refnum<vi>)
      n79 = control-ref of="CBFVBen"() -> (w102:refnum<vi>)
      n80 = control-ref of="CBFVAen"() -> (w101:refnum<vi>)
      n81 = Build Array(w69, w70, w111, w110, w109, w108, w107, w106, w105, w104, w103, w102, w101) -> (w100:refnum<vi>[])
      n82 = control-ref of="PT2FVBen"() -> (w99:refnum<vi>)
      n83 = control-ref of="PT2FVAen"() -> (w98:refnum<vi>)
      n84 = control-ref of="PT2GVPen"() -> (w97:refnum<vi>)
      n85 = control-ref of="PT1FVBen"() -> (w96:refnum<vi>)
      n86 = control-ref of="PT1FVAen"() -> (w95:refnum<vi>)
      n87 = control-ref of="PT1GVPen"() -> (w94:refnum<vi>)
      n88 = control-ref of="BOB5FVBen"() -> (w93:refnum<vi>)
      n89 = control-ref of="BOB5FVAen"() -> (w92:refnum<vi>)
      n90 = control-ref of="BOB5GVPen"() -> (w91:refnum<vi>)
      n91 = control-ref of="BOB5GVSen"() -> (w90:refnum<vi>)
      n92 = control-ref of="BOB4FVBen"() -> (w89:refnum<vi>)
      n93 = control-ref of="BOB4FVAen"() -> (w88:refnum<vi>)
      n94 = control-ref of="BOB5TPen"() -> (w79:refnum<vi>)
      n95 = Build Array (concatenate)(w100, w99, w98, w97, w96, w95, w94, w93, w92, w91, w90, w89, w88, w79) -> (w87:refnum<vi>[])
      n96 = control-ref of="BOB4GVPen"() -> (w86:refnum<vi>)
      n97 = control-ref of="BOB4GVSen"() -> (w85:refnum<vi>)
      n98 = control-ref of="BOB3FVBen"() -> (w84:refnum<vi>)
      n99 = control-ref of="BOB3FVAen"() -> (w83:refnum<vi>)
      n100 = control-ref of="BOB3GVPen"() -> (w82:refnum<vi>)
      n101 = control-ref of="BOB3GVSen"() -> (w81:refnum<vi>)
      n102 = control-ref of="BOB2TPen"() -> (w78:refnum<vi>)
      n103 = control-ref of="TSTTPen"() -> (w77:refnum<vi>)
      n104 = control-ref of="BOB3TPen"() -> (w76:refnum<vi>)
      n105 = control-ref of="CB1TPen"() -> (w75:refnum<vi>)
      n106 = control-ref of="BOB4TPen"() -> (w74:refnum<vi>)
      n107 = control-ref of="PT1TPen"() -> (w73:refnum<vi>)
      n108 = control-ref of="PT2TPen"() -> (w72:refnum<vi>)
      n109 = control-ref of="CB5GVSen"() -> (w71:refnum<vi>)
      n110 = Build Array (concatenate)(w87, w86, w85, w84, w83, w82, w81, w78, w77, w76, w75, w74, w73, w72, w71) -> (w80:refnum<vi>[])
      n111 = for "Initialize Enable Indicators" {
        tunnel: w80 -> [w113] mode=indexing
        n112 = property class="Bool (strict)"(reference=w113, "Colors [4]"=cluster{u32, u32}[] [{16711680, 16711680}, {6618880, 6618880}, {11245188, 10125428}]) -> ()  [unwired: 1 in, 2 out]
      }
    }
    frame #3 {
      # "Front Panel Indicators (Numeric)"
      n113 = control-ref of="CBLN2PIR"() -> (w141:refnum<vi>)
      n114 = control-ref of="PTLN2PIR"() -> (w140:refnum<vi>)
      n115 = control-ref of="BOB2PEN"() -> (w139:refnum<vi>)
      n116 = control-ref of="BOB2PIR"() -> (w138:refnum<vi>)
      n117 = control-ref of="BOB3PEN"() -> (w137:refnum<vi>)
      n118 = control-ref of="BOB3PIR"() -> (w136:refnum<vi>)
      n119 = control-ref of="BOB3_MCP"() -> (w135:refnum<vi>)
      n120 = control-ref of="BOB3_Pho"() -> (w134:refnum<vi>)
      n121 = control-ref of="CB1PEN"() -> (w133:refnum<vi>)
      n122 = control-ref of="CB2PEN"() -> (w132:refnum<vi>)
      n123 = control-ref of="CB3PEN"() -> (w131:refnum<vi>)
      n124 = control-ref of="BOB4PEN"() -> (w130:refnum<vi>)
      n125 = Build Array(w141, w140, w139, w138, w137, w136, w135, w134, w133, w132, w131, w130) -> (w143:refnum<vi>[])
      n126 = control-ref of="BOB4PIR"() -> (w129:refnum<vi>)
      n127 = control-ref of="BOB5PEN"() -> (w128:refnum<vi>)
      n128 = control-ref of="BOB5PIR"() -> (w127:refnum<vi>)
      n129 = control-ref of="BOB5_MCP"() -> (w126:refnum<vi>)
      n130 = control-ref of="BOB5_Pho"() -> (w125:refnum<vi>)
      n131 = control-ref of="PT1PEN"() -> (w124:refnum<vi>)
      n132 = control-ref of="PT1PIR"() -> (w123:refnum<vi>)
      n133 = control-ref of="PT2PIR"() -> (w122:refnum<vi>)
      n134 = control-ref of="PT2PEN"() -> (w117:refnum<vi>)
      n135 = control-ref of="BOB6_MCP"() -> (w118:refnum<vi>)
      n136 = control-ref of="BOB6_Pho"() -> (w119:refnum<vi>)
      n137 = control-ref of="FVBPIR"() -> (w120:refnum<vi>)
      n138 = control-ref of="FVAPIR"() -> (w121:refnum<vi>)
      n139 = control-ref of="LN2Level"() -> (w115:refnum<vi>)
      n140 = control-ref of="FVCPIR"() -> (w116:refnum<vi>)
      n141 = control-ref of="LHeLevel"() -> (w114:refnum<vi>)
      n142 = Build Array (concatenate)(w143, w129, w128, w127, w126, w125, w124, w123, w122, w117, w118, w119, w120, w121, w116, w115, w114) -> (w142:refnum<vi>[])
      n143 = for "Initialize Indicators" {
        tunnel: w142 -> [w145] mode=indexing
        n144 = property class="DigNum (strict)"(reference=w145, "Label.BG Color"=u32 16448250 ("Color Box")) -> ()  [unwired: 1 in, 2 out]
      }
    }
    frame #4 {
      n145 = control-ref of="CB5SAFE_MonData"() -> (w147:refnum<vi>)
      n146 = for "Subscribe to DIM MON Values" {
        N: 1 -> [_]
        tunnel: w147 -> [w148]
        tunnel: w147 -> [w152]
        n147 = property class="Clust (strict)"(reference=w148) -> ("Label.Text"=w151:string)  [unwired: 1 in, 2 out]
        n148 = Match Pattern(string=w151, regular expression="Data") -> (before substring=w149:string)  [unwired: 1 in, 3 out]
        n149 = call "DimIndicators.dic_info_service.vi"("controlRef"=w152, "serviceName"=w149) -> ()  [unwired: 16 in, 2 out]
      }
    }
    frame #5 {
      # "DIM Mon Values Variables (Boolean In)"
      n150 = control-ref of="BOB2TISin_MonData"() -> (w156:refnum<vi>)
      n151 = control-ref of="TSTGVSin_MonData"() -> (w199:refnum<vi>)
      n152 = control-ref of="TSTTPin_MonData"() -> (w198:refnum<vi>)
      n153 = control-ref of="TSTFVAin_MonData"() -> (w197:refnum<vi>)
      n154 = control-ref of="TSTFVBin_MonData"() -> (w196:refnum<vi>)
      n155 = control-ref of="LASFVAin_MonData"() -> (w153:refnum<vi>)
      n156 = control-ref of="LASFVBin_MonData"() -> (w154:refnum<vi>)
      n157 = control-ref of="LASGVSin_MonData"() -> (w155:refnum<vi>)
      n158 = control-ref of="BOB2FCin_MonData"() -> (w205:refnum<vi>)
      n159 = control-ref of="BOB2FVAin_MonData"() -> (w204:refnum<vi>)
      n160 = control-ref of="BOB2FVBin_MonData"() -> (w203:refnum<vi>)
      n161 = control-ref of="BOB2GVPin_MonData"() -> (w202:refnum<vi>)
      n162 = control-ref of="BOB2GVSin_MonData"() -> (w201:refnum<vi>)
      n163 = control-ref of="BOB2TPin_MonData"() -> (w200:refnum<vi>)
      n164 = Build Array(w153, w154, w155, w205, w204, w203, w202, w201, w200, w199, w198, w197, w196, w156) -> (w194:refnum<vi>[])
      n165 = control-ref of="BOB3GVSin_MonData"() -> (w195:refnum<vi>)
      n166 = control-ref of="BOB3GVPin_MonData"() -> (w193:refnum<vi>)
      n167 = control-ref of="BOB3TPin_MonData"() -> (w192:refnum<vi>)
      n168 = control-ref of="BOB3FCin_MonData"() -> (w191:refnum<vi>)
      n169 = control-ref of="BOB3MCPin_MonData"() -> (w190:refnum<vi>)
      n170 = control-ref of="BOB3FVAin_MonData"() -> (w189:refnum<vi>)
      n171 = control-ref of="BOB3FVBin_MonData"() -> (w188:refnum<vi>)
      n172 = control-ref of="CBFVAin_MonData"() -> (w187:refnum<vi>)
      n173 = control-ref of="CBFVBin_MonData"() -> (w186:refnum<vi>)
      n174 = control-ref of="CBFVCin_MonData"() -> (w185:refnum<vi>)
      n175 = control-ref of="CB1TPin_MonData"() -> (w184:refnum<vi>)
      n176 = control-ref of="CB2TPin_MonData"() -> (w183:refnum<vi>)
      n177 = control-ref of="CB3TPin_MonData"() -> (w182:refnum<vi>)
      n178 = control-ref of="CB4TPin_MonData"() -> (w181:refnum<vi>)
      n179 = control-ref of="CB5GVSin_MonData"() -> (w180:refnum<vi>)
      n180 = control-ref of="BOB4GVSin_MonData"() -> (w179:refnum<vi>)
      n181 = control-ref of="BOB4GVPin_MonData"() -> (w178:refnum<vi>)
      n182 = control-ref of="BOB4TPin_MonData"() -> (w177:refnum<vi>)
      n183 = control-ref of="BOB4BETAin_MonData"() -> (w176:refnum<vi>)
      n184 = control-ref of="BOB4FVAin_MonData"() -> (w175:refnum<vi>)
      n185 = Build Array (concatenate)(w194, w195, w193, w192, w191, w190, w189, w188, w187, w186, w185, w184, w183, w182, w181, w180, w179, w178, w177, w176, w175) -> (w174:refnum<vi>[])
      n186 = control-ref of="BOB4FVBin_MonData"() -> (w173:refnum<vi>)
      n187 = control-ref of="BOB5GVSin_MonData"() -> (w172:refnum<vi>)
      n188 = control-ref of="BOB5GVPin_MonData"() -> (w171:refnum<vi>)
      n189 = control-ref of="BOB5TPin_MonData"() -> (w170:refnum<vi>)
      n190 = control-ref of="BOB5FCin_MonData"() -> (w169:refnum<vi>)
      n191 = control-ref of="BOB5MCPin_MonData"() -> (w168:refnum<vi>)
      n192 = control-ref of="BOB5FVAin_MonData"() -> (w167:refnum<vi>)
      n193 = control-ref of="BOB5FVBin_MonData"() -> (w166:refnum<vi>)
      n194 = control-ref of="PT1GVPin_MonData"() -> (w165:refnum<vi>)
      n195 = control-ref of="PT1TPin_MonData"() -> (w164:refnum<vi>)
      n196 = control-ref of="PT1FVAin_MonData"() -> (w163:refnum<vi>)
      n197 = control-ref of="PT1FVBin_MonData"() -> (w162:refnum<vi>)
      n198 = control-ref of="PT2GVPin_MonData"() -> (w161:refnum<vi>)
      n199 = control-ref of="PT2TPin_MonData"() -> (w160:refnum<vi>)
      n200 = control-ref of="PT2FVAin_MonData"() -> (w159:refnum<vi>)
      n201 = control-ref of="PT2FVBin_MonData"() -> (w158:refnum<vi>)
      n202 = Build Array (concatenate)(w174, w173, w172, w171, w170, w169, w168, w167, w166, w165, w164, w163, w162, w161, w160, w159, w158) -> (w157:refnum<vi>[])
      n203 = for "Subscribe to DIM MON Values in" {
        tunnel: w157 -> [w206] mode=indexing
        tunnel: w157 -> [w210] mode=indexing
        n204 = property class="Clust (strict)"(reference=w206) -> ("Label.Text"=w209:string)  [unwired: 1 in, 2 out]
        n205 = Match Pattern(string=w209, regular expression="Data") -> (before substring=w207:string)  [unwired: 1 in, 3 out]
        n206 = call "DimIndicators.dic_info_service.vi"("controlRef"=w210, "serviceName"=w207) -> ()  [unwired: 16 in, 2 out]
      }
    }
    frame #6 {
      # "DIM Mon Values Variables  (Boolean Out)"
      n207 = control-ref of="TSTGVSout_MonData"() -> (w257:refnum<vi>)
      n208 = control-ref of="TSTTPout_MonData"() -> (w256:refnum<vi>)
      n209 = control-ref of="TSTFVAout_MonData"() -> (w255:refnum<vi>)
      n210 = control-ref of="TSTFVBout_MonData"() -> (w254:refnum<vi>)
      n211 = control-ref of="BOB2TISout_MonData"() -> (w214:refnum<vi>)
      n212 = control-ref of="LASFVAout_MonData"() -> (w211:refnum<vi>)
      n213 = control-ref of="LASFVBout_MonData"() -> (w212:refnum<vi>)
      n214 = control-ref of="LASGVSout_MonData"() -> (w213:refnum<vi>)
      n215 = control-ref of="BOB2FCout_MonData"() -> (w263:refnum<vi>)
      n216 = control-ref of="BOB2FVAout_MonData"() -> (w262:refnum<vi>)
      n217 = control-ref of="BOB2FVBout_MonData"() -> (w261:refnum<vi>)
      n218 = control-ref of="BOB2GVPout_MonData"() -> (w260:refnum<vi>)
      n219 = control-ref of="BOB2GVSout_MonData"() -> (w259:refnum<vi>)
      n220 = control-ref of="BOB2TPout_MonData"() -> (w258:refnum<vi>)
      n221 = Build Array(w211, w212, w213, w263, w262, w261, w260, w259, w258, w257, w256, w255, w254, w214) -> (w252:refnum<vi>[])
      n222 = control-ref of="BOB3GVSout_MonData"() -> (w253:refnum<vi>)
      n223 = control-ref of="BOB3GVPout_MonData"() -> (w251:refnum<vi>)
      n224 = control-ref of="BOB3TPout_MonData"() -> (w250:refnum<vi>)
      n225 = control-ref of="BOB3FCout_MonData"() -> (w249:refnum<vi>)
      n226 = control-ref of="BOB3MCPout_MonData"() -> (w248:refnum<vi>)
      n227 = control-ref of="BOB3FVAout_MonData"() -> (w247:refnum<vi>)
      n228 = control-ref of="BOB3FVBout_MonData"() -> (w246:refnum<vi>)
      n229 = control-ref of="CBFVAout_MonData"() -> (w245:refnum<vi>)
      n230 = control-ref of="CBFVBout_MonData"() -> (w244:refnum<vi>)
      n231 = control-ref of="CBFVCout_MonData"() -> (w243:refnum<vi>)
      n232 = control-ref of="CB1TPout_MonData"() -> (w242:refnum<vi>)
      n233 = control-ref of="CB2TPout_MonData"() -> (w241:refnum<vi>)
      n234 = control-ref of="CB3TPout_MonData"() -> (w240:refnum<vi>)
      n235 = control-ref of="CB4TPout_MonData"() -> (w239:refnum<vi>)
      n236 = control-ref of="CB5GVSout_MonData"() -> (w238:refnum<vi>)
      n237 = control-ref of="BOB4GVSout_MonData"() -> (w237:refnum<vi>)
      n238 = control-ref of="BOB4GVPout_MonData"() -> (w236:refnum<vi>)
      n239 = control-ref of="BOB4TPout_MonData"() -> (w235:refnum<vi>)
      n240 = control-ref of="BOB4BETAout_MonData"() -> (w234:refnum<vi>)
      n241 = control-ref of="BOB4FVAout_MonData"() -> (w233:refnum<vi>)
      n242 = Build Array (concatenate)(w252, w253, w251, w250, w249, w248, w247, w246, w245, w244, w243, w242, w241, w240, w239, w238, w237, w236, w235, w234, w233) -> (w232:refnum<vi>[])
      n243 = control-ref of="BOB4FVBout_MonData"() -> (w231:refnum<vi>)
      n244 = control-ref of="BOB5GVSout_MonData"() -> (w230:refnum<vi>)
      n245 = control-ref of="BOB5GVPout_MonData"() -> (w229:refnum<vi>)
      n246 = control-ref of="BOB5TPout_MonData"() -> (w228:refnum<vi>)
      n247 = control-ref of="BOB5FCout_MonData"() -> (w227:refnum<vi>)
      n248 = control-ref of="BOB5MCPout_MonData"() -> (w226:refnum<vi>)
      n249 = control-ref of="BOB5FVAout_MonData"() -> (w225:refnum<vi>)
      n250 = control-ref of="BOB5FVBout_MonData"() -> (w224:refnum<vi>)
      n251 = control-ref of="PT1GVPout_MonData"() -> (w223:refnum<vi>)
      n252 = control-ref of="PT1TPout_MonData"() -> (w222:refnum<vi>)
      n253 = control-ref of="PT1FVAout_MonData"() -> (w221:refnum<vi>)
      n254 = control-ref of="PT1FVBout_MonData"() -> (w220:refnum<vi>)
      n255 = control-ref of="PT2GVPout_MonData"() -> (w219:refnum<vi>)
      n256 = control-ref of="PT2TPout_MonData"() -> (w218:refnum<vi>)
      n257 = control-ref of="PT2FVAout_MonData"() -> (w217:refnum<vi>)
      n258 = control-ref of="PT2FVBout_MonData"() -> (w216:refnum<vi>)
      n259 = Build Array (concatenate)(w232, w231, w230, w229, w228, w227, w226, w225, w224, w223, w222, w221, w220, w219, w218, w217, w216) -> (w215:refnum<vi>[])
      n260 = for "Subscribe to DIM MON Values Out" {
        tunnel: w215 -> [w264] mode=indexing
        tunnel: w215 -> [w268] mode=indexing
        n261 = property class="Clust (strict)"(reference=w264) -> ("Label.Text"=w267:string)  [unwired: 1 in, 2 out]
        n262 = Match Pattern(string=w267, regular expression="Data") -> (before substring=w265:string)  [unwired: 1 in, 3 out]
        n263 = call "DimIndicators.dic_info_service.vi"("controlRef"=w268, "serviceName"=w265) -> ()  [unwired: 16 in, 2 out]
      }
    }
    frame #7 {
      # "DIM Set Values Variables (Boolean)"
      n264 = control-ref of="LASlock_SetData"() -> (w277:refnum<vi>)
      n265 = control-ref of="BOB2lock_SetData"() -> (w276:refnum<vi>)
      n266 = control-ref of="BOB3lock_SetData"() -> (w275:refnum<vi>)
      n267 = control-ref of="BOB4lock_SetData"() -> (w274:refnum<vi>)
      n268 = control-ref of="BOB5lock_SetData"() -> (w273:refnum<vi>)
      n269 = control-ref of="TSTlock_SetData"() -> (w272:refnum<vi>)
      n270 = control-ref of="CBlock_SetData"() -> (w271:refnum<vi>)
      n271 = control-ref of="PTlock_SetData"() -> (w270:refnum<vi>)
      n272 = Build Array(w277, w276, w275, w274, w273, w272, w271, w270) -> (w269:refnum<vi>[])
      n273 = for "Subscribe to DIM Set Values" {
        tunnel: w269 -> [w278] mode=indexing
        tunnel: w269 -> [w282] mode=indexing
        n274 = property class="Clust (strict)"(reference=w278) -> ("Label.Text"=w281:string)  [unwired: 1 in, 2 out]
        n275 = Match Pattern(string=w281, regular expression="Data") -> (before substring=w279:string)  [unwired: 1 in, 3 out]
        n276 = call "DimIndicators.dic_info_service.vi"("controlRef"=w282, "serviceName"=w279) -> ()  [unwired: 16 in, 2 out]
      }
    }
    frame #8 {
      # "DIM Monitor Values Variables (Numeric)"
      n277 = control-ref of="BOB5PEN_MonData"() -> (w290:refnum<vi>)
      n278 = control-ref of="PTLN2PIR_MonData"() -> (w296:refnum<vi>)
      n279 = control-ref of="CBLN2PIR_MonData"() -> (w297:refnum<vi>)
      n280 = control-ref of="BOB2PEN_MonData"() -> (w298:refnum<vi>)
      n281 = control-ref of="BOB2PIR_MonData"() -> (w304:refnum<vi>)
      n282 = control-ref of="BOB3PEN_MonData"() -> (w303:refnum<vi>)
      n283 = control-ref of="BOB3PIR_MonData"() -> (w312:refnum<vi>)
      n284 = control-ref of="BOB3_MCP_MonData"() -> (w311:refnum<vi>)
      n285 = control-ref of="BOB3_Pho_MonData"() -> (w310:refnum<vi>)
      n286 = control-ref of="CB1PEN_MonData"() -> (w309:refnum<vi>)
      n287 = control-ref of="CB2PEN_MonData"() -> (w308:refnum<vi>)
      n288 = control-ref of="CB3PEN_MonData"() -> (w307:refnum<vi>)
      n289 = control-ref of="BOB4PEN_MonData"() -> (w306:refnum<vi>)
      n290 = control-ref of="BOB4PIR_MonData"() -> (w305:refnum<vi>)
      n291 = control-ref of="BOB5_MCP_MonData"() -> (w292:refnum<vi>)
      n292 = control-ref of="BOB5_Pho_MonData"() -> (w291:refnum<vi>)
      n293 = control-ref of="BOB5PIR_MonData"() -> (w302:refnum<vi>)
      n294 = control-ref of="PT1PEN_MonData"() -> (w301:refnum<vi>)
      n295 = control-ref of="PT1PIR_MonData"() -> (w300:refnum<vi>)
      n296 = control-ref of="BOB6_MCP_MonData"() -> (w299:refnum<vi>)
      n297 = control-ref of="BOB6_Pho_MonData"() -> (w295:refnum<vi>)
      n298 = control-ref of="PT2PEN_MonData"() -> (w294:refnum<vi>)
      n299 = control-ref of="PT2PIR_MonData"() -> (w293:refnum<vi>)
      n300 = control-ref of="FVAPIR_MonData"() -> (w288:refnum<vi>)
      n301 = control-ref of="FVBPIR_MonData"() -> (w287:refnum<vi>)
      n302 = control-ref of="LN2Level_MonData"() -> (w285:refnum<vi>)
      n303 = control-ref of="LHeLevel_MonData"() -> (w284:refnum<vi>)
      n304 = control-ref of="FVCPIR_MonData"() -> (w283:refnum<vi>)
      n305 = Build Array(w296, w297, w298, w304, w303, w312, w311, w310, w309, w308, w307, w306, w305, w292, w291, w290) -> (w289:refnum<vi>[])
      n306 = Build Array (concatenate)(w289, w302, w301, w300, w299, w295, w294, w293, w288, w287, w285, w284, w283) -> (w286:refnum<vi>[])
      n307 = for "Subscribe to DIM  Monitor Values (Numeric)" {
        tunnel: w286 -> [w313] mode=indexing
        tunnel: w286 -> [w317] mode=indexing
        n308 = property class="Clust (strict)"(reference=w313) -> ("Label.Text"=w316:string)  [unwired: 1 in, 2 out]
        n309 = Match Pattern(string=w316, regular expression="Data") -> (before substring=w314:string)  [unwired: 1 in, 3 out]
        n310 = call "DimIndicators.dic_info_service.vi"("controlRef"=w317, "serviceName"=w314) -> ()  [unwired: 16 in, 2 out]
      }
    }
    frame #9 {
      # "Reason For Locking a section indicator and DIM variable are created here"
      # "DIM Set Values Variables"
      n311 = control-ref of="BOB5_MCP_SetData"() -> (w323:refnum<vi>)
      n312 = control-ref of="BOB6_Pho_SetData"() -> (w322:refnum<vi>)
      n313 = control-ref of="BOB6_MCP_SetData"() -> (w321:refnum<vi>)
      n314 = control-ref of="BOB3_Pho_SetData"() -> (w326:refnum<vi>)
      n315 = control-ref of="BOB3_MCP_SetData"() -> (w325:refnum<vi>)
      n316 = control-ref of="BOB5_Pho_SetData"() -> (w324:refnum<vi>)
      n317 = control-ref of="ReasonForLocking_SetData"() -> (w318:refnum<vi>)
      n318 = Build Array(w326, w325, w324, w323, w322, w321) -> (w320:refnum<vi>[])
      n319 = for "Subscribe to DIM Set Values" {
        tunnel: w320 -> [w330] mode=indexing
        n320 = property class="Clust (strict)"(reference=w330) -> ("Label.Text"=w329:string)  [unwired: 1 in, 2 out]
        n321 = Match Pattern(string=w329, regular expression="Data") -> (before substring=w327:string)  [unwired: 1 in, 3 out]
        n322 = call "DimIndicators.dic_info_service.vi"("controlRef"=w330, "serviceName"=w327) -> ()  [unwired: 16 in, 2 out]
      }
      n323 = call "DimIndicators.dic_info_service.vi"("controlRef"=w318, "serviceName"="ReasonForLocking") -> ()  [unwired: 16 in, 2 out]
    }
    frame #10 {
      # "Sort Control Arrays"
      n324 = call "SortArraysVac.vi"("EnIndicators"=w332, "DIMControSet"=w338, "DIMControlMon out"=w339, "DIMControlMon in"=w340, "FPIndicator"=w346) -> ("Boolean (Strict) (sorted)"=w331:refnum<vi>[], "DIMControSet (sorted)"=w337:refnum<vi>[], "DIMControlMon out (sorted)"=w335:refnum<vi>[], "DIMControlMon in (sorted)"=w336:refnum<vi>[], "FPIndicator sorted"=w345:refnum<vi>[])  [unwired: 17 in, 1 out]
      n325 = call "SortArraysPLC.vi"("FPIndicator in"=w344, "DIMControlMon"=w343, "DIMControSet"=w334) -> ("FPIndicator out"=w342:refnum<vi>[], "DIMControlMon out"=w341:refnum<vi>[], "DIMControSet out"=w333:refnum<vi>[])  [unwired: 20 in, 2 out]
    }
    frame #11 {
      n326 = while "Wait For User Commands and Variable Changes" {
        tunnel: w352 -> [w365]
        tunnel: w353 -> [w364]
        tunnel: w355 -> [w358]
        tunnel: w354 -> [w362]
        tunnel: w351 -> [w361]
        tunnel: w350 -> [w360]
        tunnel: w349 -> [w359]
        tunnel: w348 -> [w357]
        tunnel: w347 -> [w356]
        stop <- w366 stop-if-true
        n327 = event "Act on User Selection or Variable Changes" shown="[6] \"LASlock_SetData\", \"PTlock_SetData\", \"CBlock_SetData\", \"TSTlock_SetData\", \"BOB5lock_SetData\", \"BOB4lock_SetData\", \"BOB3lock_SetData\", \"BOB2lock_SetData\": Value Change" {
          selector: _ -> [_ _ _ _ _ _ _ _ _ _ _ _ _]
          dyn-events: _ -> [_ _ _ _ _ _ _ _ _ _ _ _ _]
          timeout: -1 -> [_ _ _ _ _ _ _ _ _ _ _ _ _]
          tunnel: [_ w367 _ _ _ _ _ _ _ _ _ _ TRUE ("stop")] -> w366
          tunnel: w365 -> [_ _ w383 w405 _ _ _ _ w531 _ _ _ w752]
          tunnel: w364 -> [_ _ w382 w404 _ _ _ _ _ w626 _ _ w753]
          tunnel: w362 -> [_ _ _ _ _ _ _ _ _ _ w722 _ w755]
          tunnel: w361 -> [_ _ w385 w410 w435 _ w469 _ _ _ _ _ w751]
          tunnel: w360 -> [_ _ w381 w408 w442 _ w471 _ w532 w628 _ _ _]
          tunnel: w359 -> [_ _ _ _ _ _ _ _ _ _ _ _ w754]
          tunnel: w358 -> [_ _ _ _ _ _ _ _ _ _ w721 _ _]
          tunnel: w357 -> [_ _ _ w413 _ _ _ _ _ _ _ _ w756]
          tunnel: w356 -> [_ _ _ _ _ _ _ _ w530 w625 _ _ _]
          event Timeout {
            # "Timeout"
            n328 = event-data() -> ()  [unwired: 1 in, 3 out]
          }
          event Menu Selection (User) {
            # "Deal With Menu Selections"
            n329 = event-data() -> ("ItemTag"=w368:string)  [unwired: 1 in]
            n330 = case "Selection?" shown="\"VacSymbols\"" w368 {
              tunnel: [_ _ _ _ TRUE ("stop")] -> w367
              frame "False", Default {
              }
              frame "Legend" {
                # "Open Legend"
                n331 = call "VacLegend.vi"("i ref in"=refnum<vi> refnum) -> ("i ref out"=→"i ref out":refnum<vi>)  [unwired: 10 in]
              }
              frame "VacSafety" {
                # "Open Vacuum Saftey Legend"
                n332 = call "VacSafety.vi"("i ref in"=refnum<vi> refnum) -> ("i ref out"=→"i ref out":refnum<vi>)  [unwired: 10 in]
              }
              frame "VacSymbols" {
                n333 = call "VacSymbols.vi"("i ref in"=refnum<vi> refnum) -> ("i ref out"=→"i ref out":refnum<vi>)  [unwired: 10 in]
              }
              frame "BUNAPP_FILE_EXIT" {
                # "Exit"
              }
            }
          }
          event "BOB6FC", "BOB3FC", "BOB2FC", "BOB5FC", "BOB4BETA", "LASGVS", "TSTGVS", "BOB2GVS", "BOB3GVS", "BOB4GVS", "BOB5GVS", "BOB2GVP", "BOB3GVP", "CB5GVS", "BOB4GVP", "BOB5GVP", "PT1GVP", "PT2GVP", "LASFVA", "LASFVB", "BOB2FVA", "BOB2FVB", "TSTFVA", "TSTFVB", "BOB3FVA", "BOB3FVB", "CBFVA", "CBFVC", "CBFVB", "BOB4FVA", "BOB4FVB", "BOB5FVA", "BOB5FVB", "PT1FVA", "PT1FVB", "PT2FVA", "PT2FVB", "BOB3TP", "TSTTP", "CB1TP", "BOB2TP", "BOB5TP", "PT2TP", "BOB4TP", "PT1TP", "BOB2TIS": Mouse Down {
            # "Find Indicator Index"
            # "Only the Prevacs, Gate Values and Turbo\npumps have enable relays"
            n334 = event-data() -> ("CtlRef"=w378:refnum<vi>)  [unwired: 1 in, 5 out]
            n335 = property class="Bool (strict)"(reference=w378) -> ("Label.Text"=w384:string)  [unwired: 1 in, 2 out]
            n336 = Search 1D Array(1D array=w381, element=w378) -> (index of element=w379:i32)  [unwired: 1 in]
            n337 = call "SectionLocked.vi"("Control Name"=w384, "DIMControSet (Locks)"=w385) -> ("Linked?"=w377:bool, "Unlocked?"=w380:bool)
            n338 = case "Section Unlocked?" shown="True" w380 {
              tunnel: w384 -> [_ w387]
              tunnel: string[] ["FVA", "FVB", "FVC", "GVP", "GVS", "TP"] -> [_ w389]
              tunnel: w383 -> [_ w392]
              tunnel: w382 -> [_ w393]
              tunnel: w379 -> [_ w391]
              tunnel: w377 -> [w386 _]
              frame False {
                # "Display Message to the User"
                n339 = call "Display Message to User"("Enable"=w386) -> ()  [unwired: 9 in, 2 out]
              }
              frame True {
                n340 = Array Size(array=w389) -> (size(s)=w388:i32)
                n341 = while "Determine if the indicator \nhas an enable relay" {
                  tunnel: w389 -> [w401] mode=indexing
                  tunnel: w387 -> [w400]
                  tunnel: [w397] -> w390
                  tunnel: w388 -> [w395]
                  i -> [w399]
                  stop <- w398 stop-if-true
                  n342 = Decrement(x=w395) -> (x-1=w394:i32)
                  n343 = Match Pattern(string=w400, regular expression=w401) -> (offset past match=w402:i32)  [unwired: 1 in, 3 out]
                  n344 = Not Equal?(x=w402, y=-1) -> (x != y?=w397:bool)
                  n345 = Equal?(x=w399, y=w394) -> (x = y?=w396:bool)
                  n346 = Or(x=w397, y=w396) -> (x .or. y?=w398:bool)
                }
                n347 = call "UpdateVacPLC.vi"("index of element"=w391, "DIMControlMon in (sorted)"=w393, "DIMControlMon out (sorted)"=w392, "Label.Text"=w387, "Enable?"=w390) -> ()  [unwired: 15 in]
              }
            }
          }
          event "BOB5MCP", "BOB3MCP", "BOB6MCP": Mouse Down {
            # "Find Indicator Index"
            n348 = event-data() -> ("CtlRef"=w407:refnum<vi>)  [unwired: 1 in, 7 out]
            n349 = property class="Bool (strict)"(reference=w407) -> ("Label.Text"=w411:string, "Value"=w414:bool)  [unwired: 1 in, 2 out]
            n350 = Search 1D Array(1D array=w408, element=w407) -> (index of element=w406:i32)  [unwired: 1 in]
            n351 = call "SectionLocked.vi"("Control Name"=w411, "DIMControSet (Locks)"=w410) -> ("Linked?"=w409:bool, "Unlocked?"=w412:bool)
            n352 = case "Section Unlocked?" shown="True" w412 {
              tunnel: w411 -> [_ w421]
              tunnel: w414 -> [_ w423]
              tunnel: w413 -> [_ w422]
              tunnel: w409 -> [w415 _]
              tunnel: w406 -> [_ w420]
              tunnel: w405 -> [_ w419]
              tunnel: w404 -> [_ w418]
              frame False {
                # "Section Locked"
                n353 = call "Display Message to User"("Enable"=w415) -> ()  [unwired: 9 in, 2 out]
              }
              frame True {
                n354 = call "CheckMCP.vi"("MCP Control Name"=w421, "MCP_DIM_SetData"=w422) -> ("No Link?"=w416:bool, "Safe?"=w417:bool)
                n355 = case "No Link?" shown="False" w416 {
                  tunnel: w423 -> [w429 _]
                  tunnel: w421 -> [w428 _]
                  tunnel: w420 -> [w427 _]
                  tunnel: w419 -> [w426 _]
                  tunnel: w418 -> [w425 _]
                  tunnel: w417 -> [w424 _]
                  frame False {
                    n356 = case "MCP Safe?" shown="True" w424 {
                      tunnel: w429 -> [_ _]
                      tunnel: w428 -> [_ w430]
                      tunnel: w427 -> [_ w433]
                      tunnel: w426 -> [_ w432]
                      tunnel: w425 -> [_ w431]
                      frame False {
                        # "MCP Not Safe"
                        n357 = call "Display Message to User"() -> ()  [unwired: 10 in, 2 out]
                      }
                      frame True {
                        # "Change MCP Position"
                        n358 = call "UpdateVacPLC.vi"("index of element"=w433, "DIMControlMon in (sorted)"=w431, "DIMControlMon out (sorted)"=w432, "Label.Text"=w430, "Enable?"=FALSE) -> ()  [unwired: 15 in]
                      }
                    }
                  }
                  frame True {
                    # "Display Message to the User"
                    n359 = call "Display Message to User"() -> ()  [unwired: 10 in, 2 out]
                  }
                }
              }
            }
          }
          event "LASlock", "BOB2lock", "CBlock", "PTlock", "BOB5lock", "BOB4lock", "BOB3lock", "TSTlock": Mouse Down; "LASlock", "BOB2lock", "TSTlock", "PTlock", "CBlock", "BOB4lock", "BOB5lock", "BOB3lock": Value Change {
            # "Find Set Index"
            n360 = event-data() -> ("CtlRef"=w443:refnum<vi>)  [unwired: 1 in]
            n361 = property class="Bool (strict)"(reference=w443) -> ("Label.Text"=w436:string)  [unwired: 1 in, 2 out]
            n362 = Search 1D Array(1D array=w442, element=w443) -> (index of element=w441:i32)  [unwired: 1 in]
            n363 = Index Array(array=w435, index=w441) -> (element=w440:refnum<vi>)
            n364 = property class="Clust (strict)"(reference=w440) -> ("Value"=w439:T8)  [unwired: 1 in, 2 out]
            n365 = Unbundle By Name(w439) -> ("no link"=w438:bool, "data"=w437:i16)
            n366 = case "No Link?" shown="False" w438 {
              tunnel: w437 -> [w449 _]
              tunnel: w436 -> [w447 _]
              frame False {
                # "Safety Overwrite Off"
                # "Update Vacuum PLC"
                n367 = Less Or Equal To 0?(x=w449) -> (x <= 0?=w448:bool)
                n368 = Boolean To (0,1)(Boolean=w448) -> (0, 1=w450:i16)
                n369 = call-poly "CoreLib.data 2 byte array.vi"("i16"=w450) -> ("byteArray out"=w445:T4)  [unwired: 18 in]
                n370 = Concatenate Strings("SetVacuum" ("string"), w447) -> (w452:string)
                n371 = call-poly "CoreLib.data 2 byte array.vi"("byteArray"=w445, "i16"=i16 0) -> ("byteArray out"=w446:T4)  [unwired: 17 in]
                n372 = Bundle By Name(cluster="call cluster in", "Object"="VacuumPLC", "Selector"=w452, "CallType"=enum16{"simple", "synchronous", "asynchronous"}."simple", "Data"=w446) -> (w455:T2)
                n373 = call "CoreLib.call process.vi"("call cluster in"=w455) -> ()  [unwired: 13 in, 2 out]
              }
              frame True {
                # "No Link"
                n374 = call "Display Message to User"() -> ()  [unwired: 10 in, 2 out]
              }
            }
          }
          event "Reason for locking": Value Change {
            # "Update Vacuum PLC"
            n375 = event-data() -> ("CtlRef"=w464:refnum<vi>)  [unwired: 1 in, 3 out]
            n376 = property class="Str"(reference=w464) -> ("Value"=w458:string)  [unwired: 1 in, 2 out]
            n377 = call "EmptyString.vi"() -> ("String"=w461:string)
            n378 = Concatenate Strings(w458, "\r\n") -> (w460:string)
            n379 = Replace Substring(4:w460, 5:w461) -> (1:w462:string)  [unwired: 2 in, 1 out]
            n380 = call-poly "CoreLib.data 2 byte array.vi"("string"=w462) -> ("byteArray out"=w457:T4)  [unwired: 18 in]
            n381 = Bundle By Name(cluster="call cluster in", "Object"="VacuumPLC", "Selector"="SetLockingReason", "CallType"=enum16{"simple", "synchronous", "asynchronous"}."simple", "Data"=w457) -> (w467:T2)
            n382 = call "CoreLib.call process.vi"("call cluster in"=w467) -> ()  [unwired: 13 in, 2 out]
          }
          event Value Change {
            n383 = event-data() -> ("CtlRef"=w470:refnum<vi>, "NewVal"=w472:T1)  [unwired: 1 in, 5 out]
            n384 = stacked-sequence "Check and update section locks" {
              tunnel: w472 -> [w475 _]
              tunnel: w471 -> [w474 _]
              tunnel: w470 -> [w473 _]
              tunnel: w469 -> [_ w497]
              frame #0 {
                n385 = for "Check if Indicator Exists for the Set Value?" {
                  tunnel: w475 -> [w484]
                  tunnel: w473 -> [w481]
                  tunnel: w474 -> [w476] mode=indexing
                  n386 = property class="Bool (strict)"(reference=w476) -> (reference out=w477:refnum<vi>, "Label.Text"=w479:string)  [unwired: 1 in, 1 out]
                  n387 = property class="Clust (strict)"(reference=w481) -> ("Label.Text"=w482:string)  [unwired: 1 in, 2 out]
                  n388 = Match Pattern(string=w482, regular expression="_SetData") -> (before substring=w478:string)  [unwired: 1 in, 3 out]
                  n389 = Equal?(x=w479, y=w478) -> (x = y?=w480:bool)
                  n390 = case "Indicator exists?" shown="True" w480 {
                    tunnel: w484 -> [w490 _]
                    tunnel: w477 -> [w489 _]
                    frame True {
                      # "Updating a Section Lock"
                      n391 = Unbundle By Name(w490) -> ("data"=w487:dbl, "no link"=w486:bool)
                      n392 = case "No Link?" shown="False" w486 {
                        tunnel: w487 -> [w492 _]
                        tunnel: [w494 FALSE] -> w488
                        tunnel: [cluster{u32, u32}[] [{1985280, 1985280}, {6618880, 6618880}, {11245188, 10125428}] ("Colors [4]") cluster{u32, u32}[] [{16448250, 16448250}, {16448250, 16448250}, {11245188, 10125428}] ("Colors [4]")] -> w485
                        frame False {
                          n393 = Equal?(x=w492, y=i16 1) -> (x = y?=w494:bool)
                        }
                        frame True {
                        }
                      }
                      n394 = property on="Property Node" class="Bool (strict)"(reference=w489, "Value"=w488, "Colors [4]"=w485) -> ()  [unwired: 1 in, 2 out]
                    }
                    frame False {
                    }
                  }
                }
              }
              frame #1 {
                # "Check if any of the sections are locked to determine if\nthe reasons for locking string should be displayed"
                n395 = for "Check if any of the sections are locked" {
                  tunnel: w497 -> [w504] mode=indexing
                  shift-right: [w503] -> w498
                  shift-left: FALSE -> [w502]
                  n396 = property class="Clust (strict)"(reference=w504) -> ("Value"=w501:T8)  [unwired: 1 in, 2 out]
                  n397 = Unbundle By Name(w501) -> ("data"=w500:i16)
                  n398 = case "Section Locked?" shown="1" w500 {
                    tunnel: w502 -> [w505 _]
                    tunnel: [w505 TRUE] -> w503
                    frame 0, Default {
                    }
                    frame 1 {
                      # "Section locked\ndisplay reasons\nfor locking"
                    }
                  }
                }
                n399 = property on="Reason for locking" class="Str"("Visible"=w498) -> ()  [unwired: 2 in, 2 out]
              }
            }
          }
          event Value Change {
            # "Get NickName"
            # "Updating a Monitor Value"
            n400 = event-data() -> ("CtlRef"=w510:refnum<vi>, "NewVal"=w511:T1)  [unwired: 1 in, 5 out]
            n401 = property class="Clust (strict)"(reference=w510) -> ("Label.Text"=w508:string)  [unwired: 1 in, 2 out]
            n402 = Match Pattern(string=w508, regular expression="_MonData") -> (before substring=w507:string)  [unwired: 1 in, 3 out]
            n403 = case "Indicator exists?" shown="\"CB5SAFE\"" w507 {
              tunnel: w511 -> [w522 _]
              frame "CB5SAFE" {
                n404 = Unbundle By Name(w522) -> ("data"=w517:dbl, "no link"=w513:bool, "quality"=w521:i32)
                n405 = Equal?(x=i16 -1, y=w517) -> (x = y?=w515:bool)
                n406 = Or(x=w515, y=w513) -> (x .or. y?=w514:bool)
                n407 = case shown="False" w513 {
                  tunnel: w521 -> [_ _]
                  tunnel: [w528 UtilityLib.valueStatus."no info available" ("valueStatus")] -> w520
                  tunnel: w517 -> [w526 _]
                  tunnel: [w527 _] -> w519
                  frame False {
                    n408 = call "CoreLib.quality 2 status.vi"("quality"=0) -> ("valueStatus"=w528:T7)  [unwired: 18 in]
                    n409 = Not Equal To 0?(x=w526) -> (x != 0?=w527:bool)
                  }
                  frame True {
                  }
                }
                n410 = case shown="False" w514 {
                  tunnel: [cluster{u32, u32}[] [{16711680, 16711680}, {6618880, 6618880}, {11245188, 10125428}] ("Colors [4]") cluster{u32, u32}[] [{16448250, 16448250}, {16448250, 16448250}, {11245188, 10125428}] ("Colors [4]")] -> w518
                  frame False {
                  }
                  frame True {
                  }
                }
                n411 = control-ref of="CB5SAFE"() -> (w512:refnum<vi>)
                n412 = property on="Property Node" class="Bool (strict)"(reference=w512, "Val(Sgnl)"=w519, "Colors [4]"=w518) -> ()  [unwired: 1 in, 2 out]
                n413 = call "TextColor(bool).vi"("valueStatus"=w520, "Ref"=w512) -> ()  [unwired: 10 in]
              }
              frame Default {
              }
            }
          }
          event Value Change {
            n414 = event-data() -> ("CtlRef"=w533:refnum<vi>, "NewVal"=w534:T1)  [unwired: 1 in, 5 out]
            n415 = for "Check if Indicator Exists for the Monitor Value?" {
              tunnel: w534 -> [w550]
              tunnel: w533 -> [w547]
              tunnel: w532 -> [w544] mode=indexing
              tunnel: w531 -> [w543]
              tunnel: w530 -> [w540]
              i -> [w538]
              # "Updating a Monitor Value"
              n416 = property class="Bool (strict)"(reference=w544) -> (reference out=w535:refnum<vi>, "Label.Text"=w537:string)  [unwired: 1 in, 1 out]
              n417 = property class="Clust (strict)"(reference=w547) -> ("Label.Text"=w548:string)  [unwired: 1 in, 2 out]
              n418 = Index Array(array=w540, index=w538) -> (element=w539:refnum<vi>)
              n419 = Index Array(array=w543, index=w538) -> (element=w542:refnum<vi>)
              n420 = property class="Clust (strict)"(reference=w542) -> ("Value"=w541:T8)  [unwired: 1 in, 2 out]
              n421 = Match Pattern(string=w548, regular expression="in_MonData") -> (before substring=w545:string)  [unwired: 1 in, 3 out]
              n422 = Equal?(x=w537, y=w545) -> (x = y?=w546:bool)
              n423 = case "Indicator exists?" shown="True" w546 {
                tunnel: w550 -> [w572 _]
                tunnel: w535 -> [w570 _]
                tunnel: w541 -> [w569 _]
                tunnel: w539 -> [w557 _]
                tunnel: w537 -> [w552 _]
                tunnel: string[] ["FC", "MCP", "BETA", "TIS"] -> [w553 _]
                frame True {
                  n424 = Unbundle By Name(w569) -> ("data"=w561:i16, "no link"=w566:bool, "quality"=w565:i32)
                  n425 = Unbundle By Name(w572) -> ("data"=w562:dbl, "no link"=w567:bool, "quality"=w558:i32)
                  n426 = while "Is a Detector?" {
                    tunnel: w553 -> [w580] mode=indexing
                    tunnel: w552 -> [w581]
                    tunnel: [w573] -> w551
                    i -> [w579]
                    stop <- w575 stop-if-true
                    n427 = Match Pattern(string=w581, regular expression=w580) -> (offset past match=w577:i32)  [unwired: 1 in, 3 out]
                    n428 = Equal?(x=w579, y=3) -> (x = y?=w574:bool)
                    n429 = Not Equal?(x=-1, y=w577) -> (x != y?=w573:bool)
                    n430 = Or(x=w573, y=w574) -> (x .or. y?=w575:bool)
                  }
                  n431 = Multiply(x=i16 2, y=w561) -> (x*y=w560:i16)
                  n432 = Or(x=w566, y=w567) -> (x .or. y?=w568:bool)
                  n433 = Add(x=w560, y=w562) -> (x+y=w563:dbl)
                  n434 = case "No Link to DIM?" shown="False" w568 {
                    tunnel: [w583 UtilityLib.valueStatus."no info available" ("valueStatus")] -> w571
                    tunnel: [w589 cluster{u32, u32}[] [{16448250, 16448250}, {16448250, 16448250}, {11245188, 10125428}] ("Colors [4]")] -> w564
                    tunnel: w565 -> [w585 _]
                    tunnel: w563 -> [w588 _]
                    tunnel: [w587 w622] -> w559
                    tunnel: [w586 w622] -> w555
                    tunnel: w558 -> [w584 _]
                    tunnel: w551 -> [w582 _]
                    frame False {
                      n435 = case "Act on Monitors?" shown="1" w588 {
                        tunnel: [cluster{u32, u32}[] [{16776960, 16776960}, {16776960, 16776960}, {11245188, 10125428}] ("Colors [4]") w601 w605 cluster{u32, u32}[] [{16711680, 16711680}, {16711680, 16711680}, {11245188, 10125428}] ("Colors [4]") cluster{u32, u32}[] [{16448250, 16448250}, {16448250, 16448250}, {11245188, 10125428}] ("Colors [4]")] -> w589
                        tunnel: [FALSE TRUE FALSE FALSE w620] -> w587
                        tunnel: [TRUE w596 w606 TRUE w620] -> w586
                        tunnel: w585 -> [_ w598 _ _ _]
                        tunnel: w584 -> [w591 _ w607 w614 w618]
                        tunnel: [w592 w599 w608 w615 w619] -> w583
                        tunnel: w582 -> [_ w595 w604 _ _]
                        frame 0 {
                          # "In - False  Out - False"
                          n436 = call "CoreLib.quality 2 status.vi"("quality"=w591) -> ("valueStatus"=w592:T7)  [unwired: 18 in]
                        }
                        frame 1 {
                          # "In - True  Out - False"
                          n437 = case "Is a Detector?" shown="False" w595 {
                            tunnel: [cluster{u32, u32}[] [{6618880, 6618880}, {1985280, 1985280}, {11245188, 10125428}] ("Colors [4]") cluster{u32, u32}[] [{1985280, 1985280}, {6618880, 6618880}, {11245188, 10125428}] ("Colors [4]")] -> w601
                            frame False {
                            }
                            frame True {
                            }
                          }
                          n438 = Equal?(x=w598, y=3) -> (x = y?=w596:bool)
                          n439 = call "CoreLib.quality 2 status.vi"("quality"=w598) -> ("valueStatus"=w599:T7)  [unwired: 18 in]
                        }
                        frame 2 {
                          # "In - False  Out - True"
                          n440 = case "Is a Detector?" shown="True" w604 {
                            tunnel: [cluster{u32, u32}[] [{6618880, 6618880}, {1985280, 1985280}, {11245188, 10125428}] ("Colors [4]") cluster{u32, u32}[] [{1985280, 1985280}, {6618880, 6618880}, {11245188, 10125428}] ("Colors [4]")] -> w605
                            frame False {
                            }
                            frame True {
                            }
                          }
                          n441 = call "CoreLib.quality 2 status.vi"("quality"=w607) -> ("valueStatus"=w608:T7)  [unwired: 18 in]
                          n442 = Equal?(x=w607, y=3) -> (x = y?=w606:bool)
                        }
                        frame 3 {
                          # "In - True  Out - True"
                          n443 = call "CoreLib.quality 2 status.vi"("quality"=w614) -> ("valueStatus"=w615:T7)  [unwired: 18 in]
                        }
                        frame -2, -1, Default {
                          w620 = FALSE
                          # "No Link to DIM"
                          n444 = call "CoreLib.quality 2 status.vi"("quality"=w618) -> ("valueStatus"=w619:T7)  [unwired: 18 in]
                        }
                      }
                    }
                    frame True {
                      w622 = FALSE
                      # "No Link to DIM"
                    }
                  }
                  n445 = Not(x=w555) -> (.not. x?=w556:bool)
                  n446 = property on="Property Node" class="Bool (strict)"(reference=w570, "Colors [4]"=w564, "Val(Sgnl)"=w559) -> ()  [unwired: 1 in, 2 out]
                  n447 = property on="Property Node" class="Bool (strict)"(reference=w557, "Value"=w556) -> ()  [unwired: 1 in, 2 out]
                  n448 = call "TextColor(bool).vi"("valueStatus"=w571, "Ref"=w570) -> ()  [unwired: 10 in]
                }
                frame False {
                }
              }
            }
          }
          event Value Change {
            n449 = event-data() -> ("CtlRef"=w627:refnum<vi>, "NewVal"=w629:T1)  [unwired: 1 in, 5 out]
            n450 = for "Check if Indicator Exists for the Monitor Value?" {
              tunnel: w629 -> [w645]
              tunnel: w627 -> [w642]
              tunnel: w628 -> [w638] mode=indexing
              tunnel: w626 -> [w637]
              tunnel: w625 -> [w632]
              i -> [w634]
              # "Updating a Monitor Value"
              n451 = property class="Bool (strict)"(reference=w638) -> (reference out=w639:refnum<vi>, "Label.Text"=w631:string)  [unwired: 1 in, 1 out]
              n452 = property class="Clust (strict)"(reference=w642) -> ("Label.Text"=w643:string)  [unwired: 1 in, 2 out]
              n453 = Index Array(array=w637, index=w634) -> (element=w636:refnum<vi>)
              n454 = Index Array(array=w632, index=w634) -> (element=w633:refnum<vi>)
              n455 = property class="Clust (strict)"(reference=w636) -> ("Value"=w635:T8)  [unwired: 1 in, 2 out]
              n456 = Match Pattern(string=w643, regular expression="out_MonData") -> (before substring=w640:string)  [unwired: 1 in, 3 out]
              n457 = Equal?(x=w631, y=w640) -> (x = y?=w641:bool)
              n458 = case "Indicator exists?" shown="True" w641 {
                tunnel: w645 -> [w655 _]
                tunnel: w639 -> [w657 _]
                tunnel: w635 -> [w656 _]
                tunnel: w633 -> [w649 _]
                tunnel: w631 -> [w648 _]
                tunnel: string[] ["FC", "MCP", "BETA", "TIS"] -> [w647 _]
                frame True {
                  n459 = Unbundle By Name(w656) -> ("data"=w654:i16, "no link"=w661:bool, "quality"=w662:i32)
                  n460 = Unbundle By Name(w655) -> ("data"=w653:dbl, "no link"=w660:bool, "quality"=w667:i32)
                  n461 = while "Is a Detector?" {
                    tunnel: w647 -> [w675] mode=indexing
                    tunnel: w648 -> [w676]
                    tunnel: [w668] -> w646
                    i -> [w674]
                    stop <- w670 stop-if-true
                    n462 = Match Pattern(string=w676, regular expression=w675) -> (offset past match=w672:i32)  [unwired: 1 in, 3 out]
                    n463 = Equal?(x=w674, y=3) -> (x = y?=w669:bool)
                    n464 = Not Equal?(x=-1, y=w672) -> (x != y?=w668:bool)
                    n465 = Or(x=w668, y=w669) -> (x .or. y?=w670:bool)
                  }
                  n466 = Multiply(x=i16 2, y=w653) -> (x*y=w652:dbl)
                  n467 = Or(x=w661, y=w660) -> (x .or. y?=w659:bool)
                  n468 = Add(x=w654, y=w652) -> (x+y=w664:dbl)
                  n469 = case "No Link to DIM?" shown="False" w659 {
                    tunnel: [w678 UtilityLib.valueStatus."no info available" ("valueStatus")] -> w658
                    tunnel: [w684 cluster{u32, u32}[] [{16448250, 16448250}, {16448250, 16448250}, {11245188, 10125428}] ("Colors [4]")] -> w663
                    tunnel: w662 -> [w680 _]
                    tunnel: w664 -> [w683 _]
                    tunnel: [w682 w717] -> w666
                    tunnel: [w681 w717] -> w650
                    tunnel: w667 -> [w679 _]
                    tunnel: w646 -> [w677 _]
                    frame False {
                      n470 = case "Act on Monitors?" shown="-2, -1, Default" w683 {
                        tunnel: [cluster{u32, u32}[] [{16776960, 16776960}, {16776960, 16776960}, {11245188, 10125428}] ("Colors [4]") w691 w700 cluster{u32, u32}[] [{16711680, 16711680}, {16711680, 16711680}, {11245188, 10125428}] ("Colors [4]") cluster{u32, u32}[] [{16448250, 16448250}, {16448250, 16448250}, {11245188, 10125428}] ("Colors [4]")] -> w684
                        tunnel: [FALSE TRUE FALSE FALSE w715] -> w682
                        tunnel: [TRUE w694 w702 TRUE w715] -> w681
                        tunnel: w680 -> [_ _ w701 _ _]
                        tunnel: w679 -> [w686 w692 _ w709 w713]
                        tunnel: [w687 w695 w703 w710 w714] -> w678
                        tunnel: w677 -> [_ w690 w699 _ _]
                        frame 0 {
                          # "In - False  Out - False"
                          n471 = call "CoreLib.quality 2 status.vi"("quality"=w686) -> ("valueStatus"=w687:T7)  [unwired: 18 in]
                        }
                        frame 1 {
                          # "In - True  Out - False"
                          n472 = case "Is a Detector?" shown="False" w690 {
                            tunnel: [cluster{u32, u32}[] [{6618880, 6618880}, {1985280, 1985280}, {11245188, 10125428}] ("Colors [4]") cluster{u32, u32}[] [{1985280, 1985280}, {6618880, 6618880}, {11245188, 10125428}] ("Colors [4]")] -> w691
                            frame False {
                            }
                            frame True {
                            }
                          }
                          n473 = Equal?(x=w692, y=3) -> (x = y?=w694:bool)
                          n474 = call "CoreLib.quality 2 status.vi"("quality"=w692) -> ("valueStatus"=w695:T7)  [unwired: 18 in]
                        }
                        frame 2 {
                          # "In - False  Out - True"
                          n475 = case "Is a Detector?" shown="False" w699 {
                            tunnel: [cluster{u32, u32}[] [{6618880, 6618880}, {1985280, 1985280}, {11245188, 10125428}] ("Colors [4]") cluster{u32, u32}[] [{1985280, 1985280}, {6618880, 6618880}, {11245188, 10125428}] ("Colors [4]")] -> w700
                            frame False {
                            }
                            frame True {
                            }
                          }
                          n476 = call "CoreLib.quality 2 status.vi"("quality"=w701) -> ("valueStatus"=w703:T7)  [unwired: 18 in]
                          n477 = Equal?(x=w701, y=3) -> (x = y?=w702:bool)
                        }
                        frame 3 {
                          # "In - True  Out - True"
                          n478 = call "CoreLib.quality 2 status.vi"("quality"=w709) -> ("valueStatus"=w710:T7)  [unwired: 18 in]
                        }
                        frame -2, -1, Default {
                          w715 = FALSE
                          # "No Link to DIM"
                          n479 = call "CoreLib.quality 2 status.vi"("quality"=w713) -> ("valueStatus"=w714:T7)  [unwired: 18 in]
                        }
                      }
                    }
                    frame True {
                      w717 = FALSE
                      # "No Link to DIM"
                    }
                  }
                  n480 = Not(x=w650) -> (.not. x?=w651:bool)
                  n481 = property on="Property Node" class="Bool (strict)"(reference=w657, "Colors [4]"=w663, "Val(Sgnl)"=w666) -> ()  [unwired: 1 in, 2 out]
                  n482 = property on="Property Node" class="Bool (strict)"(reference=w649, "Value"=w651) -> ()  [unwired: 1 in, 2 out]
                  n483 = call "TextColor(bool).vi"("valueStatus"=w658, "Ref"=w657) -> ()  [unwired: 10 in]
                }
                frame False {
                }
              }
            }
          }
          event Value Change {
            # "Find Monitor Index"
            # "Updating a Numeric Monitor Value"
            n484 = event-data() -> ("CtlRef"=w723:refnum<vi>, "NewVal"=w724:T1)  [unwired: 1 in]
            n485 = Search 1D Array(1D array=w722, element=w723) -> (index of element=w726:i32)  [unwired: 1 in]
            n486 = Index Array(array=w721, index=w726) -> (element=w720:refnum<vi>)
            n487 = Not A Number/Path/Refnum?(number/path/refnum=w720) -> (NaN/Path/Refnum?=w725:bool)
            n488 = case "Indicator exists?" shown="False" w725 {
              tunnel: w724 -> [_ w733]
              tunnel: w720 -> [_ w727]
              frame True {
              }
              frame False {
                n489 = Unbundle By Name(w733) -> ("data"=w729:dbl, "no link"=w730:bool, "quality"=w732:i32)
                n490 = case "No Link?" shown="False" w730 {
                  tunnel: w732 -> [w736 _]
                  tunnel: [w735 UtilityLib.valueStatus."no info available" ("valueStatus")] -> w731
                  tunnel: w729 -> [w734 _]
                  tunnel: [w734 inf] -> w728
                  frame False {
                    n491 = call "CoreLib.quality 2 status.vi"("quality"=w736) -> ("valueStatus"=w735:T7)  [unwired: 18 in]
                  }
                  frame True {
                  }
                }
                n492 = property class="DigNum (strict)"(reference=w727, "Value"=w728) -> ()  [unwired: 1 in, 2 out]
                n493 = call "TextColor.vi"("valueStatus"=w731, "reference"=w727) -> ()  [unwired: 10 in]
              }
            }
          }
          event Value Change {
            # "Update Reason For Locking Indicator"
            n494 = event-data() -> ("NewVal"=w739:T5)  [unwired: 1 in]
            n495 = Unbundle By Name(w739) -> ("data"=w743:string, "no link"=w742:bool, "quality"=w741:i32)
            n496 = case "No Link?" shown="False" w742 {
              tunnel: w741 -> [w748 _]
              tunnel: [w747 UtilityLib.valueStatus."no info available" ("valueStatus")] -> w745
              tunnel: w743 -> [w746 _]
              tunnel: [w746 w749] -> w744
              frame False {
                n497 = call "CoreLib.quality 2 status.vi"("quality"=w748) -> ("valueStatus"=w747:T7)  [unwired: 18 in]
              }
              frame True {
                n498 = call "EmptyString.vi"() -> ("String"=w749:string)
              }
            }
            n499 = control-ref of="Reason for locking"() -> (w740:refnum<vi>)
            n500 = property class="Str"(reference=w740, "Value"=w744) -> ()  [unwired: 1 in, 2 out]
            n501 = call "UtilityLib.set color of GUI object.vi"("GUI object Ref"=w740, "valueStatus"=w745) -> ()  [unwired: 17 in, 1 out]
          }
          event Panel Close? {
            n502 = event-data() -> ()  [unwired: 1 in, 4 out]
            n503 = stacked-sequence {
              tunnel: w756 -> [w765 _]
              tunnel: w755 -> [w764 _]
              tunnel: w754 -> [w759 _]
              tunnel: w753 -> [w763 _]
              tunnel: w752 -> [w762 _]
              tunnel: w751 -> [w761 _]
              frame #0 {
                # "Release DIM Services"
                n504 = for "For Each Service" {
                  tunnel: w763 -> [w767] mode=indexing
                  n505 = Not A Number/Path/Refnum?(number/path/refnum=w767) -> (NaN/Path/Refnum?=w766:bool)
                  n506 = case "Not a Reference?" shown="False" w766 {
                    tunnel: w767 -> [w768 _]
                    frame False {
                      n507 = call "DimIndicators.dic_release_service.vi"("controlRef"=w768) -> ()  [unwired: 18 in, 1 out]
                    }
                    frame True {
                    }
                  }
                }
                n508 = for "For Each Service" {
                  tunnel: w761 -> [w773] mode=indexing
                  n509 = Not A Number/Path/Refnum?(number/path/refnum=w773) -> (NaN/Path/Refnum?=w772:bool)
                  n510 = case "Not a Reference?" shown="False" w772 {
                    tunnel: w773 -> [w774 _]
                    frame False {
                      n511 = call "DimIndicators.dic_release_service.vi"("controlRef"=w774) -> ()  [unwired: 18 in, 1 out]
                    }
                    frame True {
                    }
                  }
                }
                n512 = for "For Each Service" {
                  tunnel: w764 -> [w770] mode=indexing
                  n513 = Not A Number/Path/Refnum?(number/path/refnum=w770) -> (NaN/Path/Refnum?=w769:bool)
                  n514 = case "Not a Reference?" shown="False" w769 {
                    tunnel: w770 -> [w771 _]
                    frame False {
                      n515 = call "DimIndicators.dic_release_service.vi"("controlRef"=w771) -> ()  [unwired: 18 in, 1 out]
                    }
                    frame True {
                    }
                  }
                }
                n516 = control-ref of="ReasonForLocking_SetData"() -> (w760:refnum<vi>)
                n517 = for "For Each Service" {
                  tunnel: w765 -> [w782] mode=indexing
                  n518 = Not A Number/Path/Refnum?(number/path/refnum=w782) -> (NaN/Path/Refnum?=w781:bool)
                  n519 = case "Not a Reference?" shown="False" w781 {
                    tunnel: w782 -> [w783 _]
                    frame False {
                      n520 = call "DimIndicators.dic_release_service.vi"("controlRef"=w783) -> ()  [unwired: 18 in, 1 out]
                    }
                    frame True {
                    }
                  }
                }
                n521 = for "For Each Service" {
                  N: 1 -> [_]
                  tunnel: w759 -> [w779]
                  n522 = Not A Number/Path/Refnum?(number/path/refnum=w779) -> (NaN/Path/Refnum?=w778:bool)
                  n523 = case "Not a Reference?" shown="False" w778 {
                    tunnel: w779 -> [w780 _]
                    frame False {
                      n524 = call "DimIndicators.dic_release_service.vi"("controlRef"=w780) -> ()  [unwired: 18 in, 1 out]
                    }
                    frame True {
                    }
                  }
                }
                n525 = for "For Each Service" {
                  tunnel: w762 -> [w776] mode=indexing
                  n526 = Not A Number/Path/Refnum?(number/path/refnum=w776) -> (NaN/Path/Refnum?=w775:bool)
                  n527 = case "Not a Reference?" shown="False" w775 {
                    tunnel: w776 -> [w777 _]
                    frame False {
                      n528 = call "DimIndicators.dic_release_service.vi"("controlRef"=w777) -> ()  [unwired: 18 in, 1 out]
                    }
                    frame True {
                    }
                  }
                }
                n529 = call "DimIndicators.dic_release_service.vi"("controlRef"=w760) -> ()  [unwired: 18 in, 1 out]
              }
              frame #1 {
                # "Close Front Panel"
                n530 = Current VI's Path() -> (path=w787:path)
                n531 = Open VI Reference(vi path=w787) -> (vi reference=w785:refnum<vi>, error out=w784:errorcluster)  [unwired: 5 in]
                n532 = property class="VI"(reference=w785, error in=w784, "Front Panel Window:Open"=FALSE) -> ()  [unwired: 2 out]
              }
            }
            n533 = event-data() -> ()  [unwired: 2 in, 1 out]
          }
        }
      }
    }
    frame #12 {
      n534 = stacked-sequence "Release DIM Variables" {
        tunnel: w792 -> [w799 _ _]
        tunnel: w793 -> [w800 _ _]
        tunnel: w791 -> [w798 _ _]
        tunnel: w790 -> [w797 _ _]
        tunnel: w789 -> [w801 _ _]
        tunnel: w788 -> [w795 _ _]
        frame #0 {
          # "Release DIM Services"
          n535 = for "For Each Service" {
            tunnel: w799 -> [w803] mode=indexing
            n536 = Not A Number/Path/Refnum?(number/path/refnum=w803) -> (NaN/Path/Refnum?=w802:bool)
            n537 = case "Not a Reference?" shown="False" w802 {
              tunnel: w803 -> [w804 _]
              frame False {
                n538 = call "DimIndicators.dic_release_service.vi"("controlRef"=w804) -> ()  [unwired: 18 in, 1 out]
              }
              frame True {
              }
            }
          }
          n539 = for "For Each Service" {
            tunnel: w797 -> [w809] mode=indexing
            n540 = Not A Number/Path/Refnum?(number/path/refnum=w809) -> (NaN/Path/Refnum?=w808:bool)
            n541 = case "Not a Reference?" shown="False" w808 {
              tunnel: w809 -> [w810 _]
              frame False {
                n542 = call "DimIndicators.dic_release_service.vi"("controlRef"=w810) -> ()  [unwired: 18 in, 1 out]
              }
              frame True {
              }
            }
          }
          n543 = for "For Each Service" {
            tunnel: w800 -> [w806] mode=indexing
            n544 = Not A Number/Path/Refnum?(number/path/refnum=w806) -> (NaN/Path/Refnum?=w805:bool)
            n545 = case "Not a Reference?" shown="False" w805 {
              tunnel: w806 -> [w807 _]
              frame False {
                n546 = call "DimIndicators.dic_release_service.vi"("controlRef"=w807) -> ()  [unwired: 18 in, 1 out]
              }
              frame True {
              }
            }
          }
          n547 = control-ref of="ReasonForLocking_SetData"() -> (w796:refnum<vi>)
          n548 = call "DimIndicators.dic_release_service.vi"("controlRef"=w796) -> ()  [unwired: 18 in, 1 out]
          n549 = for "For Each Service" {
            tunnel: w801 -> [w818] mode=indexing
            n550 = Not A Number/Path/Refnum?(number/path/refnum=w818) -> (NaN/Path/Refnum?=w817:bool)
            n551 = case "Not a Reference?" shown="False" w817 {
              tunnel: w818 -> [w819 _]
              frame False {
                n552 = call "DimIndicators.dic_release_service.vi"("controlRef"=w819) -> ()  [unwired: 18 in, 1 out]
              }
              frame True {
              }
            }
          }
          n553 = for "For Each Service" {
            N: 1 -> [_]
            tunnel: w795 -> [w815]
            n554 = Not A Number/Path/Refnum?(number/path/refnum=w815) -> (NaN/Path/Refnum?=w814:bool)
            n555 = case "Not a Reference?" shown="False" w814 {
              tunnel: w815 -> [w816 _]
              frame False {
                n556 = call "DimIndicators.dic_release_service.vi"("controlRef"=w816) -> ()  [unwired: 18 in, 1 out]
              }
              frame True {
              }
            }
          }
          n557 = for "For Each Service" {
            tunnel: w798 -> [w812] mode=indexing
            n558 = Not A Number/Path/Refnum?(number/path/refnum=w812) -> (NaN/Path/Refnum?=w811:bool)
            n559 = case "Not a Reference?" shown="False" w811 {
              tunnel: w812 -> [w813 _]
              frame False {
                n560 = call "DimIndicators.dic_release_service.vi"("controlRef"=w813) -> ()  [unwired: 18 in, 1 out]
              }
              frame True {
              }
            }
          }
        }
        frame #1 {
          # "Close Front Panel"
          n561 = Current VI's Path() -> (path=w823:path)
          n562 = Open VI Reference(vi path=w823) -> (vi reference=w821:refnum<vi>, error out=w820:errorcluster)  [unwired: 5 in]
          n563 = property class="VI"(reference=w821, error in=w820, "Front Panel Window:Open"=FALSE) -> ()  [unwired: 2 out]
        }
        frame #2 {
          # "Stop Panel"
          n564 = Stop(stop? (T)=TRUE) -> ()
        }
      }
    }
  }
  n565 = call "LVDimInterface.dim_operate.vi"("DNSNode"="lebit-balcony") -> ()  [unwired: 19 in]
